vi "SEC code V4.9.vi"() -> ()   [LabVIEW 2022 SP3]
uses:
  SEC code V3.1/Drivers and Aux files/user.lib/atmcd32d.llb/Shutter_type typedef.ctl
  C:/SEC Software V4.91/EcoChemie.Autolab.Sdk.dll
  EcoChemie.Autolab.Sdk.dll
  SEC code V3.1/Drivers and Aux files/State.ctl
  SEC code V3.1/Drivers and Aux files/SECenumctl.ctl
  SEC code V3.1/Drivers and Aux files/user.lib/atmcd32d.llb/TriggerMode_mode typedef.ctl
  SEC code V3.1/Drivers and Aux files/OSSPEC.ctl
  SEC code V3.1/Drivers and Aux files/OSPEC-enum.ctl
  Labview/IVIUM/IVIUM_remdriver.lvlib
panel:
  out "Current PD 2":dbl
  out "POtential PD 2":dbl
  in  "Tab Control 5":enum32{"AUTOLAB", "IVIUM", "iDUS", "Kymera"}(tab)
  out "current":dbl
  out "Error after autolab connection?":errorcluster
  out "Autolab Connected?":bool
  out "Voltage":dbl format="%#_3e"
  out "PotentialOverload":bool
  out "Bandwidth":i32
  out "CurrentRange":i32
  out "Mode":i32
  out "Measured voltage":dbl
  out "CurrentOverload":bool
  out "Cell on?":bool
  out "current":dbl caption="Current (A)" format="%_4g"
  out "cell on":bool
  out "V (during measurment)":dbl
  out "Potentiostat Status":string
  out "T reached?":bool
  out "Shut down sequence run?":bool
  out "Curent Temp":i32
  in  "Tab Control 4":T1(tab)
  in  "Use autolab?":bool=TRUE
  in  "Embedded Exe File":path=path "C:/Program Files/Metrohm Autolab/Autolab SDK 2.1/Hardware Setup Files/Adk.x"
  in  "Hardware Setup File":path=path "C:/ProgramData/Metrohm Autolab/13.0/HardwareSetup.AUT55444.xml"
  in  "Bandwidth 2":i32(ring)=2 items=["UltraHigh_Speed", "High_Speed", "High_Stability"]
  in  "Start potential (V)":dbl=0.2
  in  "Stop potential (V)":dbl=0.7
  in  "Increment (V)":dbl=0.05
  in  "Default Potential (V)":dbl=0.2
  in  "Wait before \nspectrum (s)":dbl=0.1
  in  "Equilibration \ntime (s)":u32=5
  in  "Reverse Scan\ndirection":bool
  in  "(update and read)":bool
  in  "Tab Control 3":T2(tab)=enum."iDUS run"
  in  "Inetegration\n Time (us)":i32=8000
  in  "Continuous \nStrobe Delay (us)":i32
  in  "Number of averages":i32
  in  "Use iDus?":bool
  in  "Return detector \nto room T?":bool
  in  "Init, Cool, read dark,\nOR\nWarm/de-init detector":bool
  in  "Temperature\n(degrees C)":i32=-80
  in  "Number of scans in kinetic cycle":i32=30
  in  "Exposure time (s)":dbl=0.03
  in  "Tab Control 2":T3(tab)
  in  "V 1 time (s)":dbl=10.0
  in  "V off time":dbl=30.0
  in  "Sampling\n delay (s)":dbl
  in  "V 2 time (s)":dbl=20.0
  in  "Run OSPSEC":bool
  in  "Square wave?":bool
  out "OCP I (close to 0)":dbl
  out "OCP":dbl format="%_3f"
  in  "V1 (V)":dbl=0.4
  in  "V2 (V)":dbl=0.8
  in  "Slow sample time (s)":dbl=1500.0
  out "Time during PD":u32
  in  "File Name":string="test-1"
  in  "File Path":path=path "C:/Data"
  in  "Tab Control":T4(tab)
  out "?":T5(graph)
  out "?":cluster{i32[], dbl[]}(graph)
  out "?":T5(graph)
  out "?":T5(graph)
  out "Current during PD":dbl(graph)=1.602783203125e-06
  out "?":cluster{dbl[], dbl[]}(graph)
  out "Potential  During PD":dbl(graph)=-0.0002471923828124972
  out "Setpoint":dbl
  out "?":cluster{i32[], "array":i32[]}(graph)
  out "I_overload":bool
  out "Aninput1_overload":bool
  out "E_overload":bool
  out "cell-off button pressed":bool
  in  "Default\nCurrent range":T6(ring)=enum."100 uA"
  in  "Default Filter":T7(ring)=enum."10 kHz"
  out "Device serial number":string
  in  "Set Stability":T8(ring)=enum."Standard"
  out "Number of Spectrometers":i32
  out "IDus not in read loop? (kinetic)":bool
  out "Get status return code":dbl
  out "xpixels":i32
  out "ypixels":i32
  out "Calculated exposure time":sgl format="%.2f"
  out "Check timings return code":u32
  out "Set temprature\nreturn code":u32
  out "get aquired data return code":u32
  out "Start Aquisition return code":u32
  out "Init. return code":u32
  out "Cooler Off return code":u32
  out "Time before the start of current aquisition (ms)":u32
  out "Time  after the aquisition (before fetch data), (ms)":u32
  in  "Shutter opens on TTL":T9=enum."TTL High"
  in  "Shutter open and close time":i32
  out "Get aqisition ok? (kinetic mode)":bool
  out "Time taken to apply V2":u32
  out "Values to re-intialise to at end\nof the measument":T10
  out "V2 applied?":bool
  out "ContinuousStrobe Out":u32
  out "Wrapper Out":u32
  out "WL Values":dbl[](array[numeric])
  out "Number of time the OCEAN averaging loop has run -1":i32
  out "Adc":refnum<k24>
  out "Sampler 2":refnum<k24>
  out "Dio":refnum<k24>
  out "Dac":refnum<k24>
  out "instrument":refnum<k24>
  out "Ei":refnum<k24>
  out "AutolabConnection":refnum<k24>
  out "EI status supported for":string[](array[string])
  out "TemperatureOverload":bool
  out "ManualCellSwitch":bool
  out "Oscillation":bool
  out "PD ENDED\nEXIT MEASURMENT":bool=TRUE
  out "Current PD":dbl
  out "POtential PD":dbl
  in  "Exit and disconnect":bool
  # "Program control"
  # "Potential decay control"
  # "Spectrometer control"
  # "System status"
  # "SEC control"
  # "Cell on?"
  # "Use the integration time program in the same folder as this program\nto get the optimum value. For kinetic mode the time resolution is limited \nby integration time"
  # "Unless you know what you are doing keep these at 0.03 and 30"
  # "I overload overload"
  # "off button pressed"
  # "Aninput1 overload"
  # "E overload"
  # "OSPEC loop exit"
  # "Checklist for avoiding errors:\n(1) Light on the IVIUM should be blue with red flashes\nIf the system crahes and the light is red then connect and disconnect in IVUM soft/turn stat off/on\n(2) Maya Pro should read in ocean view/or the get intensity program\nIf maya is not reading connect and disconnect USB.\n(3) If errors persist rrepeat steps 1 + 2 then re-compile code by clicking the\nwhite (run) whilst holding down CRTL + (left) SHIFT\n(4) IF USING THE iDus DO NOT EXIT WITHOUT WARMING CAMERA BACK TO ROOM T,YOU \nWILL DAMAGE IT \n(6) if the IVIUM.dll does not load click broken arrows and \"show error\" until you see the call library function (see blue circles). Double click on this and paste the following into the directory (red circle):   \n%windir%\\Labview\\IVIUM\\IVIUM_remdriver.dll"
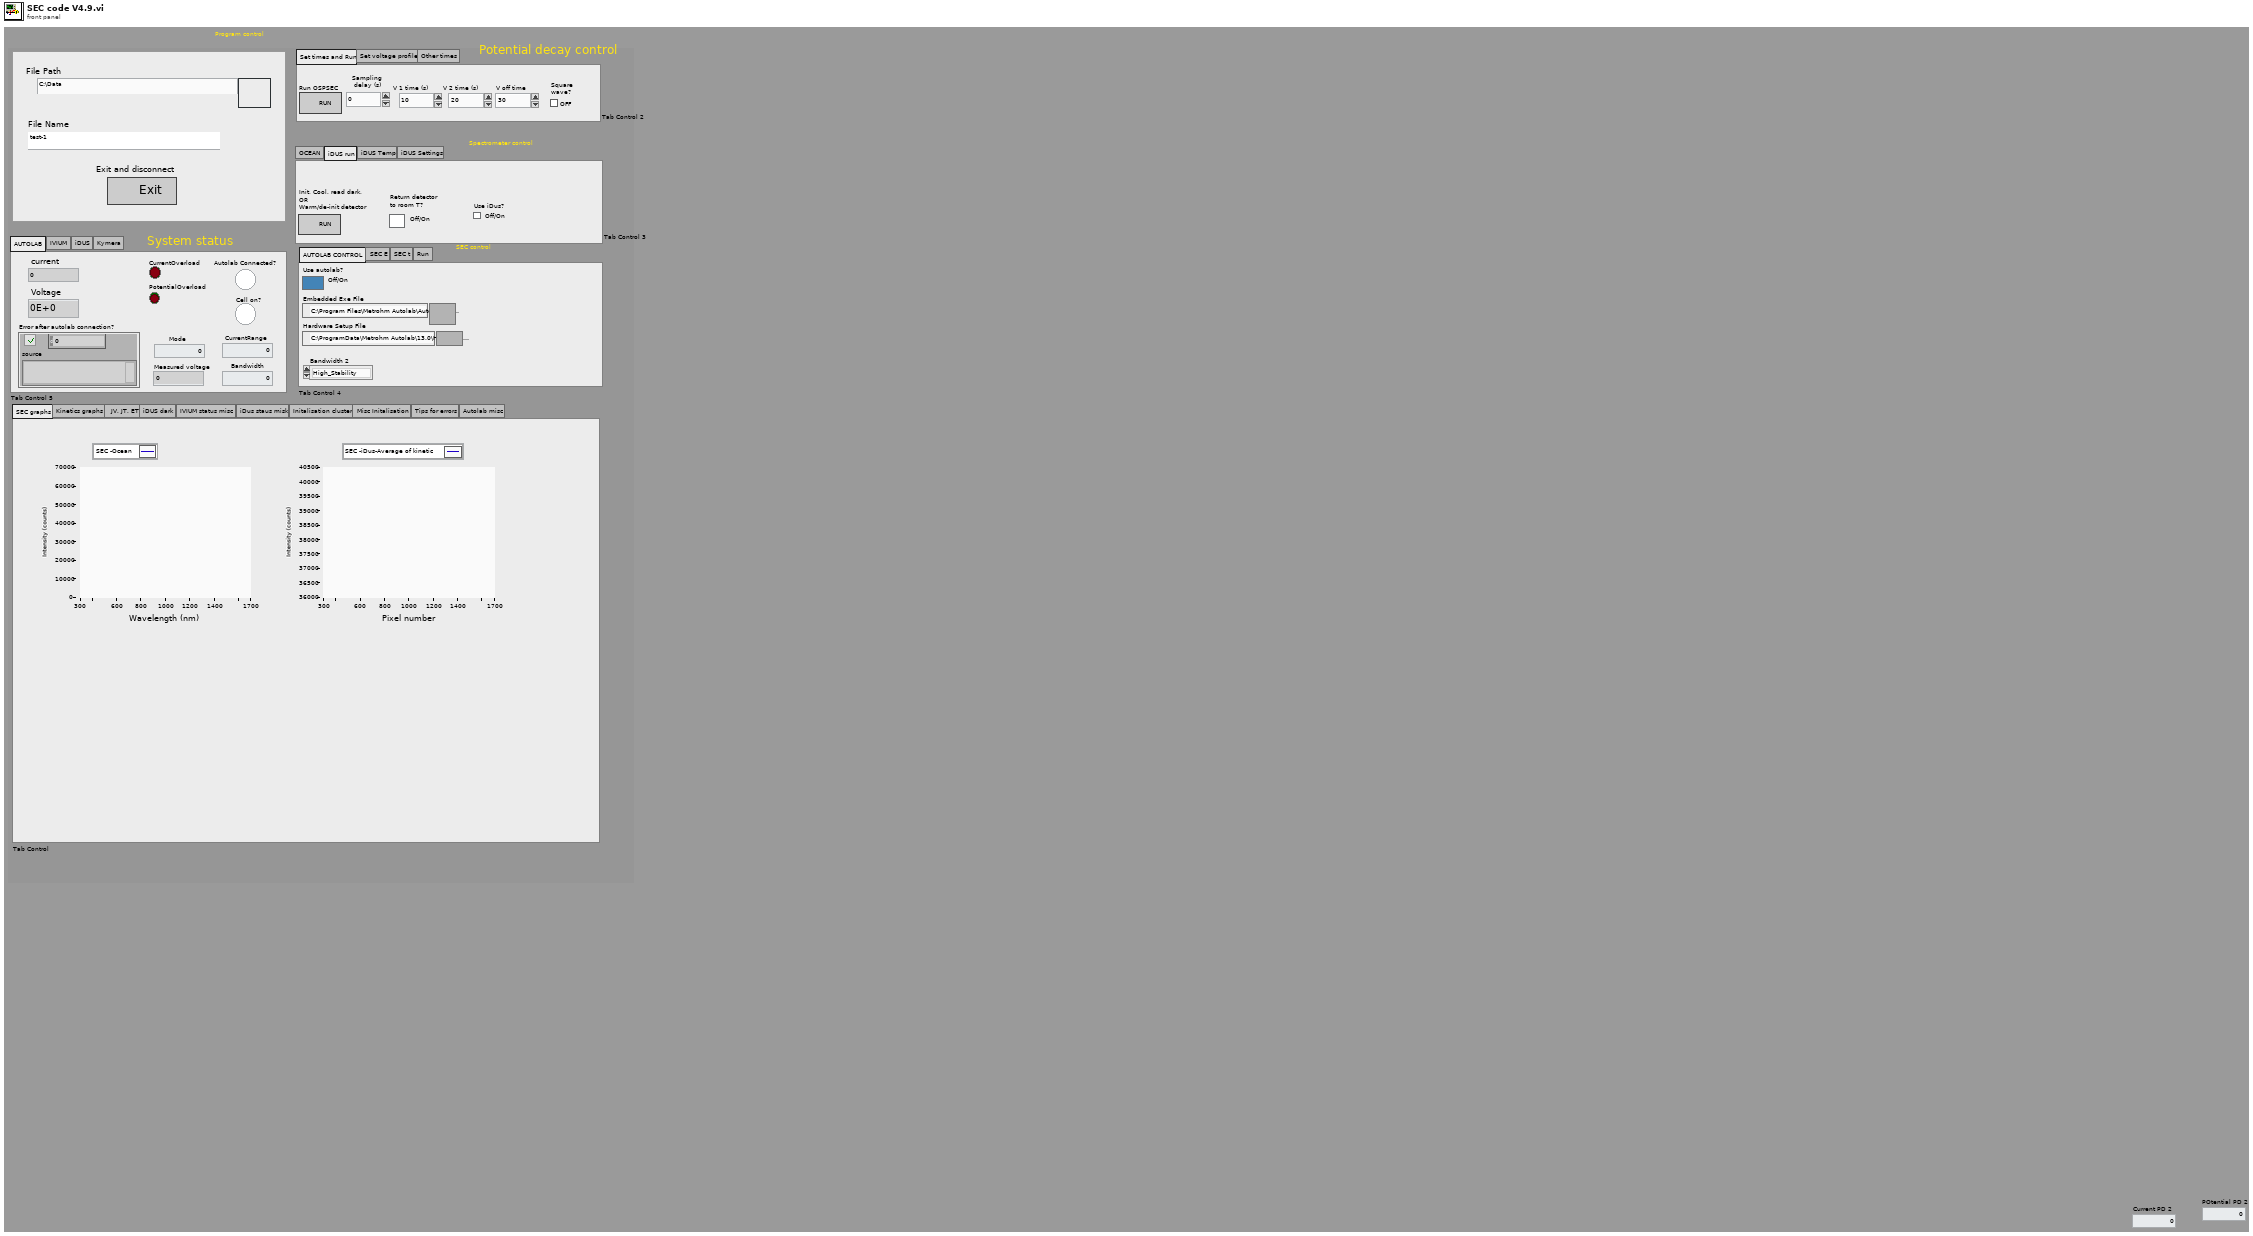
[diagram p1: front panel]
types:
  T1 = enum32{"AUTOLAB CONTROL", "SEC E", "SEC t", "Run"}
  T2 = enum32{"OCEAN", "iDUS run", "iDUS Temp", "iDUS Settings"}
  T3 = enum32{"Set times and Run", "Set voltage profile", "Other times"}
  T4 = enum32{"SEC graphs", "Kinetics graphs", " JV, JT, ET", "iDUS dark", "IVIUM status misc", "iDus staus misk", "Initalisation cluster", "Misc Initalisation ", "Tips for errors", "Autolab misc"}
  T5 = cluster{"WL Values":dbl[], "Spectrum Values":dbl[]}
  T6 = enum16{"10 A", "1 A", "100 mA", "10 mA", "1 mA", "100 uA", "10 uA", "1 uA", "100 nA", "10 nA", "1 nA", "100 pA", "10 pA", "1 pA"}
  T7 = enum16{"1 MHz", "100 kHz", "10 kHz", "1 kHz", "10 Hz"}
  T8 = enum16{"High Speed", "Standard", "High Stability"}
  T9 = typedef "Shutter_type typedef.ctl" = enum16{"TTL Low", "TTL High"}
  T10 = cluster{"Currents":dbl[], "Potentials":dbl[], "Device Status":string, "Device serial no":string, "Current":dbl, "Default \nPotential":dbl, "I overload":bool, "Cell On":bool, "E overload":bool, "Aninput1 overload":bool, "Cell off button pressed":bool, "Start potential":dbl, "Stop potential":dbl, "Increment":dbl, "SEC":dbl[], "Path":path, "File name":string}
  T11 = cluster{"Current array":dbl[], "Potential array":dbl[], "Status":string, "Serial No":string, "Current":dbl, "Default\n potential":dbl, "I overload":bool, "Cell on":bool, "E overload":bool, "Cell of button pressed":bool, "Aninput1 overload":bool, "Stop \npotential":dbl, "Start \npotential":dbl, "Increment":dbl, "Spectrum":dbl[][], "Path":path, "File Name":string, "Sample rate":dbl, "V2 time":dbl, "V off time":dbl, "V 2":dbl, "V 1":dbl, "V1 time":dbl, "Time array":dbl[], "Integration time":i32, "Continous strobe delay":i32, "Time elapsed ":i32, "Start time":i32, "Time for E measurment":i32[], "Time for I measurment ":i32[], "Time for spectrum measurment":i32[], "Return detector to \nroom T":bool, "Number of scans in kinetic cycle":i32, "Exposure time":dbl}
  T12 = typedef "State.ctl" = enum16{"Initialize", "Wait for Event", "Run SEC", "Run OSPEC", "Initialse and cool iDus", "Exit"}
  T13 = typedef "SECenumctl.ctl" = enum16{"Read spectrum from Ocean", "Read spectrum from iDus", "Apply potential", "Wait", "Apply potential Autolab"}
  T14 = typedef "TriggerMode_mode typedef.ctl" = enum16{"Internal", "External", "N/A (2)", "N/A (3)", "N/A (4)", "N/A (5)", "External Start", "External Exposure (Bulb)", "N/A (8)", "External FVB EM", "Software", "N/A (11)", "External Charge Shifting"}
  T15 = typedef "OSSPEC.ctl" = enum16{"Read Potential and spectrum", "Read current and spectrum", "Reinitialise Cell", "Apply V1", "End measurment", "Apply V2"}
  T16 = typedef "OSPEC-enum.ctl" = enum16{"Check exit", "Read", "Wait"}
  T17 = enum16{"off", "EStat4EL", "EStat2EL", "EStatDummy1", "EStatDummy2", "EStatDummy3", "EStatDummy4", "IStat4EL", "IStat2EL", "IStatDummy", "BiStat4EL", "BiStat2EL"}
  T18 = cluster{"Current array":dbl[], "Potential array":dbl[], "Status":string, "Serial No":string, "Current":dbl, "Default\n potential":dbl, "I overload":bool, "Cell on":bool, "E overload":bool, "Cell of button pressed":bool, "Aninput1 overload":bool, "Stop \npotential":dbl, "Start \npotential":dbl, "Increment":dbl, "Spectrum":dbl[][], "Path":path, "File Name":string, "Sample rate":dbl, "V2 time":dbl, "V off time":dbl, "V 2":dbl, "V 1":dbl, "V1 time":dbl, "Time array":dbl[], "Integration time":i32, "Continous strobe delay":i32, "Time elapsed ":i32, "Start time":i32, "Time for E measurment":i32[], "Time for I measurment ":i32[], "Time for spectrum measurment":i32[], "Return detector to \nroom T":bool, "Number of scans in kinetic cycle":i32, "Exposure time":i32}
  T19 = typedef "Error Code Enum typedef.ctl" = enum32{"N/A (0)", "DRV_ERROR_CODES", "DRV_SUCCESS", "DRV_VXDNOTINSTALLED", "DRV_ERROR_SCAN", "DRV_ERROR_CHECK_SUM", "DRV_ERROR_FILELOAD", "DRV_UNKNOWN_FUNC", "DRV_ERROR_VXD_INIT", "DRV_ERROR_ADDRESS", "DRV_ERROR_PAGELOCK", "DRV_ERROR_PAGEUNLOCK", "DRV_ERROR_BOARDTEST", "DRV_ERROR_ACK", "DRV_ERROR_UP_FIFO", "DRV_ERROR_PATTERN", "N/A (16)", "DRV_ACQUISITION_ERRORS", "DRV_ACQ_BUFFER", "DRV_ACQ_DOWNFIFO_FULL", "DRV_PROC_UNKONWN_INSTRUCTION", "DRV_ILLEGAL_OP_CODE", "DRV_KINETIC_TIME_NOT_MET", "DRV_ACCUM_TIME_NOT_MET", "DRV_NO_NEW_DATA", "N/A (25)", "DRV_SPOOLERROR", "N/A (27)", "N/A (28)", "N/A (29)", "N/A (30)", "N/A (31)", "N/A (32)", "DRV_TEMPERATURE_CODES", "DRV_TEMPERATURE_OFF", "DRV_TEMPERATURE_NOT_STABILIZED", "DRV_TEMPERATURE_STABILIZED", "DRV_TEMPERATURE_NOT_REACHED", "DRV_TEMPERATURE_OUT_RANGE", "DRV_TEMPERATURE_NOT_SUPPORTED", "DRV_TEMPERATURE_DRIFT", "N/A (41)", "N/A (42)", "N/A (43)", "N/A (44)", "N/A (45)", "N/A (46)", "N/A (47)", "N/A (48)", "DRV_GENERAL_ERRORS", "DRV_INVALID_AUX", "DRV_COF_NOTLOADED", "DRV_FPGAPROG", "DRV_FLEXERROR", "DRV_GPIBERROR", "N/A (55)", "N/A (56)", "N/A (57)", "N/A (58)", "N/A (59)", "N/A (60)", "N/A (61)", "N/A (62)", "N/A (63)", "DRV_DATATYPE", "DRV_DRIVER_ERRORS", "DRV_P1INVALID", "DRV_P2INVALID", "DRV_P3INVALID", "DRV_P4INVALID", "DRV_INIERROR", "DRV_COFERROR", "DRV_ACQUIRING", "DRV_IDLE", "DRV_TEMPCYCLE", "DRV_NOT_INITIALIZED", "DRV_P5INVALID", "DRV_P6INVALID", "DRV_INVALID_MODE", "DRV_INVALID_FILTER", "DRV_I2CERRORS", "DRV_I2CDEVNOTFOUND", "DRV_I2CTIMEOUT", "DRV_P7INVALID", "N/A (84)", "N/A (85)", "N/A (86)", "N/A (87)", "N/A (88)", "N/A (89)", "DRV_IOCERROR", "DRV_VRMVERSIONERROR"}
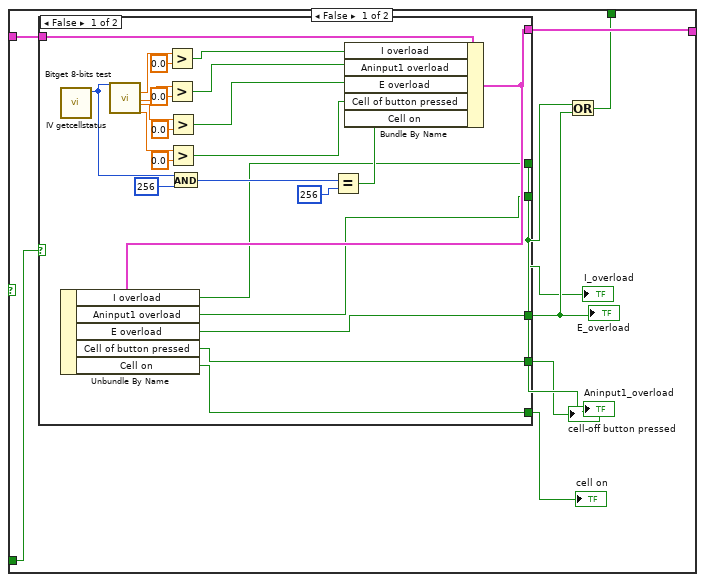
[diagram p2: hidden frame]
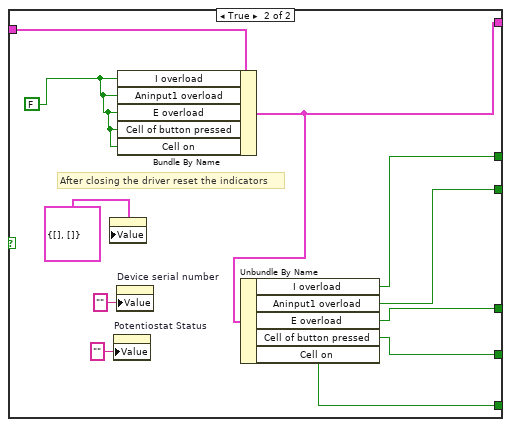
[diagram p3: hidden frame]
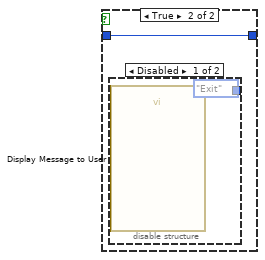
[diagram p4: hidden frame]
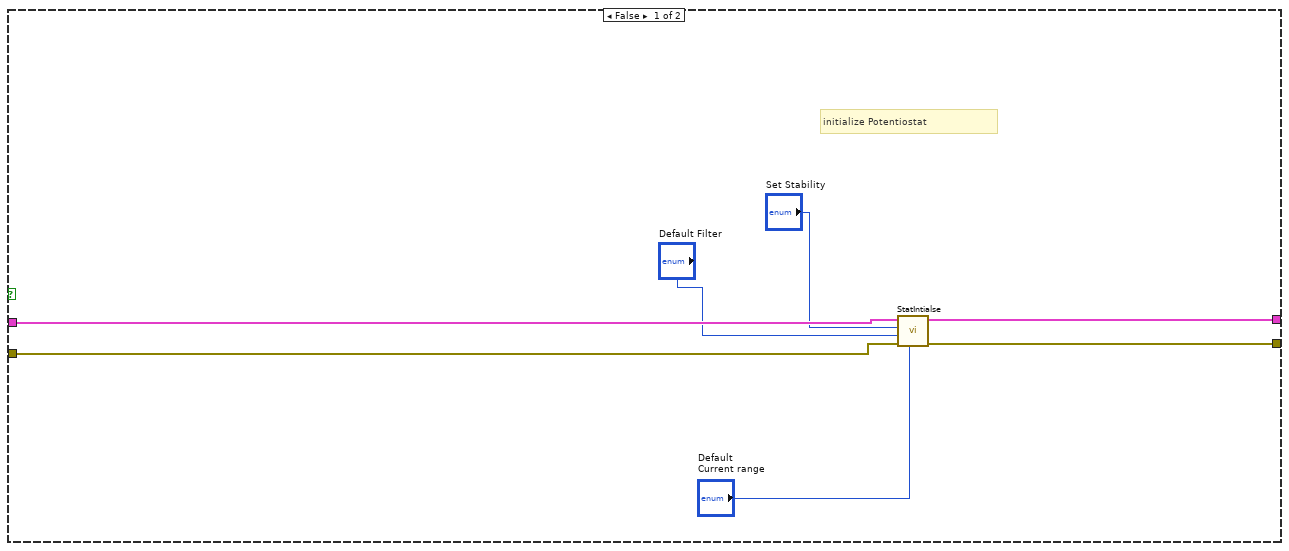
[diagram p7: hidden frame]
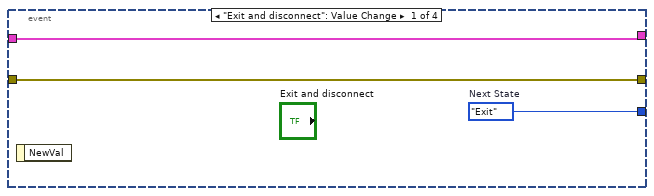
[diagram p9: hidden frame]
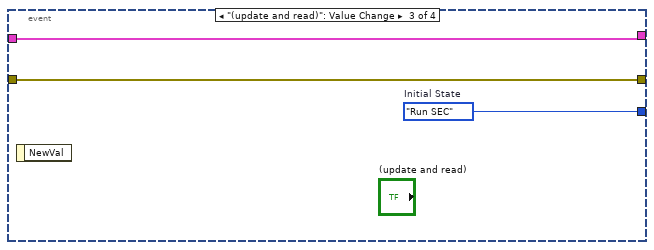
[diagram p10: hidden frame]
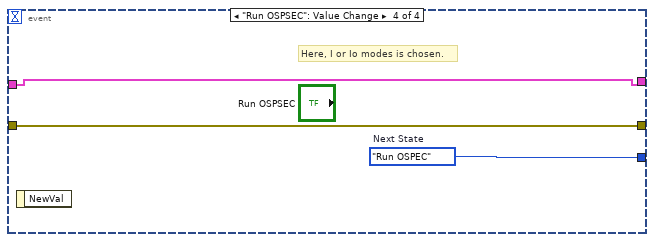
[diagram p11: hidden frame]
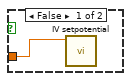
[diagram p13: hidden frame]
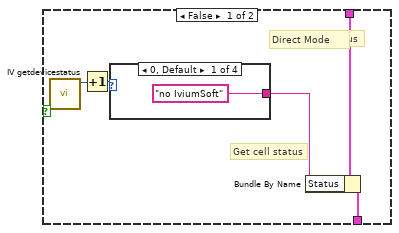
[diagram p14: hidden frame]
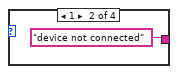
[diagram p15: hidden frame]
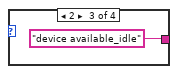
[diagram p16: hidden frame]
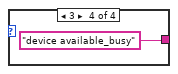
[diagram p17: hidden frame]
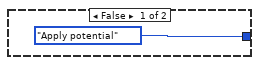
[diagram p18: hidden frame]
diagram:
  w1 = T11 {"Current array"=[], "Potential array"=[], "Status"="", "Serial No"="", "Current"=0.0, "Default\n potential"=0.0, "I overload"=FALSE, "Cell on"=FALSE, "E overload"=FALSE, "Cell of button pressed"=FALSE, "Aninput1 overload"=FALSE, "Stop \npotential"=0.0, "Start \npotential"=0.0, "Increment"=0.0, "Spectrum"=[], "Path"=path "", "File Name"="", "Sample rate"=0.0, "V2 time"=0.0, "V off time"=0.0, "V 2"=0.0, "V 1"=0.0, "V1 time"=0.0, "Time array"=[], "Integration time"=0, "Continous strobe delay"=0, "Time elapsed "=0, "Start time"=0, "Time for E measurment"=[], "Time for I measurment "=[], "Time for spectrum measurment"=[], "Return detector to \nroom T"=FALSE, "Number of scans in kinetic cycle"=0, "Exposure time"=0.0}  # Init cluster
  w3 = State."Initialize"  # Initial State
  n1 = while {
    shift-right: [w21] -> _
    shift-left: w3 -> [w38]
    shift-right: [w24] -> _
    shift-left: w1 -> [w17]
    shift-right: [w25] -> _
    shift-left: errorcluster {"status"=FALSE, "code"=0, "source"=""} ("error constant") -> [w37]
    stop <- w35 stop-if-true
    # "Main VI State Machine"
    n2 = Bundle By Name(cluster=w17, "Sample rate"="Sampling\n delay (s)", "V1 time"="V 1 time (s)", "V2 time"="V 2 time (s)", "V off time"="V off time", "V 2"="V2 (V)", "V 1"="V1 (V)", "Integration time"="Inetegration\n Time (us)", "Continous strobe delay"="Continuous \nStrobe Delay (us)", "Exposure time"="Exposure time (s)", "Number of scans in kinetic cycle"="Number of scans in kinetic cycle") -> (w11:T11)
    n3 = Bundle By Name(cluster=w11, "Default\n potential"="Default Potential (V)", "Start \npotential"="Start potential (V)", "Stop \npotential"="Stop potential (V)", "Increment"="Increment (V)", "Path"="File Path", "File Name"="File Name") -> (w23:T11)
    n4 = case shown="\"Run OSPEC\"" w38 {
      tunnel: [w94 w137 w185 w506 w546 w1742] -> w7
      tunnel: [w93 w134 FALSE ("Stop Loop?") w503 FALSE ("Stop Loop?") _] -> w36
      tunnel: w23 -> [w91 w131 w174 w507 w545 w1740]
      tunnel: [w90 w132 w159 w507 w541 w1740] -> w31
      tunnel: w37 -> [w95 w136 w183 w509 w543 w1739]
      tunnel: [w96 w135 w182 w510 w542 w1739] -> w25
      tunnel: [1 ("devconnect") 1 ("devconnect") 1 ("devconnect") w508 1 ("devconnect") 1 ("devconnect")] -> w22
      frame "Initialize" {
        w93 = FALSE  # Stop Loop?
        w94 = State."Wait for Event"  # Next State
        # "Initialize - Initialize variables needed"
        n5 = case shown="True" "Use autolab?" {
          tunnel: [w104 w109] -> w96
          tunnel: w95 -> [w103 _]
          tunnel: w91 -> [w102 w111]
          tunnel: [w98 w111] -> w90
          frame False {
            # "initialize Potentiostat"
            n6 = call "StatIntialse.vi"("Init cluster 2"=w102, "Set Stability"="Set Stability", "Default\n Filter"="Default Filter", "error in (no error)"=w103, "Default\nCurrent range"="Default\nCurrent range") -> ("Init cluster"=w98:T18, "error out"=w104:errorcluster)  [unwired: 4 in]
          }
          frame True {
            w108 = 2 items=["UltraHigh_Speed", "High_Speed", "High_Stability"] ("Bandwidth")
            w113 = 0 items=["Potentiostatic", "Galvanostatic"] ("Mode")
            w114 = -4 items=["CR07_1A"=0, "CR06_10A"=1, "CR01_100A"=2, "CR00_1000A"=3, "CR05_20A"=20, "CR04_40A"=40, "CR03_50A"=60, "CR02_80A"=80, "CR19_1pA"=-12, "CR18_10pA"=-11, "CR17_100pA"=-10, "CR16_1nA"=-9, "CR15_10nA"=-8, "CR14_100nA"=-7, "CR13_1uA"=-6, "CR12_10uA"=-5, "CR11_100uA"=-4, "CR10_1mA"=-3, "CR09_10mA"=-2, "CR08_100mA"=-1] ("CurrentRange")
            w115 = 1 items=["Off", "On"] ("CellOnOff")
            n7 = call "Connect AutoLab.vi"("Embedded Exe File"="Embedded Exe File", "Hardware Setup File"="Hardware Setup File") -> ("error out"=w120:errorcluster, ".NET Refnum out"=w129:refnum<k24>)  [unwired: 8 in]
            "Error after autolab connection?" <- w120
            n8 = property class="Instrument"(reference=w129, error in=w120) -> (reference out=→"instrument":refnum<k24>, error out=w121:errorcluster, "Adc"=→"Adc":refnum<k24>, "Dac"=→"Dac":refnum<k24>, "Dio"=→"Dio":refnum<k24>, "AutolabConnection"=w117:refnum<k24>, "Ei"=w107:refnum<k24>)
            "AutolabConnection" <- w117
            n9 = property class="AutolabConnection"(reference=w117) -> ("IsConnected"=→"Autolab Connected?":bool)  [unwired: 1 in, 2 out]
            n10 = property class="EI"(reference=w107, error in=w121) -> (reference out=→"Ei":refnum<k24>, error out=w128:errorcluster, "Sampler"=→"Sampler 2":refnum<k24>)
            n11 = Unbundle By Name(w111) -> ("Default\n potential"=w110:dbl)
            n12 = Build Array(w121, w128) -> (w122:errorcluster[])
            n13 = Merge Errors(w122) -> (w112:errorcluster)
            n14 = property class="EI" props=["Bandwidth", "CellOnOff", "CurrentRange", "Mode", "Setpoint", "Current", "Potential", "PotentialApplied", "PotentialOverload", "Sampler", "Setpoint", "PotentialOverload"](reference=w107, error in=w112, "Bandwidth"=w108, "CellOnOff"=w115, "CurrentRange"=w114, "Mode"=w113, "Setpoint"=w110) -> (error out=w109:errorcluster)  [unwired: 8 out]
            n15 = property class="EI"(reference=w107) -> ("Potential"=w106:dbl, "Current"=w105:dbl)  [unwired: 1 in, 2 out]
            n16 = property on="current" class="DigNum (strict)"("Value"=w105) -> ()  [unwired: 2 in, 2 out]
            n17 = property on="Voltage" class="DigNum (strict)"("Value"=w106) -> ()  [unwired: 2 in, 2 out]
          }
        }
        n18 = property on="V2 applied?" class="Bool (strict)"("Value"=FALSE ("V2 applied")) -> ()  [unwired: 2 in, 2 out]
        "Values to re-intialise to at end\nof the measument" <- T10 {"Currents"=[], "Potentials"=[], "Device Status"="", "Device serial no"="", "Current"=0.0, "Default \nPotential"=0.0, "I overload"=FALSE, "Cell On"=FALSE, "E overload"=FALSE, "Aninput1 overload"=FALSE, "Cell off button pressed"=FALSE, "Start potential"=0.0, "Stop potential"=0.0, "Increment"=0.0, "SEC"=[], "Path"=path "", "File name"=""} ("Values to re-intialise to at end\nof the measument")
      }
      frame "Wait for Event" {
        w134 = FALSE  # Stop Loop?
        # "Wait for Event - Use an Event Structure to monitor the user interface for events that run different states of the state machine."
        n19 = event shown="[1] \"Init, Cool, read dark, OR Warm/de-init detector\": Value Change" {
          selector: _ -> [_ _ _ _]
          dyn-events: _ -> [_ _ _ _]
          timeout: _ -> [_ _ _ _]
          tunnel: [w140 State."Initialse and cool iDus" ("Next State") w147 w151] -> w137
          tunnel: w136 -> [w139 w145 w148 w150]
          tunnel: [w139 w145 w148 w150] -> w135
          tunnel: w131 -> [w138 w143 w146 w149]
          tunnel: [w138 w141 w146 w149] -> w132
          event "Exit and disconnect": Value Change {
            w140 = State."Exit"  # Next State
            n20 = event-data() -> ()  [unwired: 1 in, 1 out]
          }
          event "Init, Cool, read dark,\nOR\nWarm/de-init detector": Value Change {
            n21 = event-data() -> ()  [unwired: 1 in, 4 out]
            n22 = Bundle By Name(cluster=w143, "Return detector to \nroom T"="Return detector \nto room T?") -> (w141:T11)
          }
          event "(update and read)": Value Change {
            w147 = State."Run SEC"  # Initial State
            n23 = event-data() -> ()  [unwired: 1 in, 1 out]
          }
          event "Run OSPSEC": Value Change {
            w151 = State."Run OSPEC"  # Next State
            # "Here, I or Io modes is chosen."
            n24 = event-data() -> ()  [unwired: 1 in, 1 out]
          }
        }
      }
      frame "Run SEC" {
        w185 = State."Wait for Event"  # Next State
        n25 = property on="Use autolab?" class="Bool (strict)"() -> ("Value"=w154:bool)  [unwired: 2 in, 2 out]
        n26 = case shown="True" w154 {
          tunnel: w174 -> [w191 w199]
          tunnel: [w190 w199] -> w161
          frame False {
            # "Get cell status"
            # "Get Device Status"
            # "Direct Mode"
            n27 = call "IV getdevicestatus.vi"() -> ("return type"=w193:i32)  [unwired: 10 in, 1 out]
            n28 = Increment(x=w193) -> (x+1=w192:i32)
            n29 = case shown="0, Default" w192 {
              tunnel: ["no IviumSoft" "device not connected" "device available_idle" "device available_busy"] -> w194
              frame 0, Default {
              }
              frame 1 {
              }
              frame 2 {
              }
              frame 3 {
              }
            }
            n30 = Bundle By Name(cluster=w191, "Status"=w194) -> (w190:T11)
          }
          frame True {
          }
        }
        n31 = property on="Use autolab?" class="Bool (strict)"() -> ("Value"=w156:bool)  [unwired: 2 in, 2 out]
        n32 = case shown="True" w156 {
          tunnel: [SECenumctl."Apply potential" SECenumctl."Apply potential Autolab"] -> w181
          frame False {
          }
          frame True {
          }
        }
        n33 = Unbundle By Name(w161) -> ("Increment"=w180:dbl, "Start \npotential"=w184:dbl, "Stop \npotential"=w175:dbl)
        n34 = while {
          shift-right: [w227] -> w158
          shift-left: w161 -> [w228]
          tunnel: w180 -> [w223]
          tunnel: w184 -> [w222]
          shift-right: [w224] -> w182
          shift-left: w183 -> [w225]
          shift-right: [w216] -> _
          shift-left: w181 -> [w220]
          shift-right: [w218] -> w160
          shift-left: dbl[] [0.0] -> [w217]
          shift-right: [w213] -> w164
          shift-left: dbl[] [0.0] -> [w214]
          tunnel: w175 -> [w215]
          shift-right: [w212] -> w173
          shift-left: dbl[][] [] -> [w211]
          tunnel: "Reverse Scan\ndirection" -> [w210]
          tunnel: [w208] -> _
          tunnel: [w208] -> _
          shift-right: [w207] -> _
          shift-left: -3 ("y") -> [w206]
          i -> [w226]
          stop <- w208 stop-if-true
          n35 = case shown="\"Read spectrum from Ocean\"" w220 {
            tunnel: w228 -> [w251 w315 w350 w365 w465]
            tunnel: [w250 w314 w350 w365 w465] -> w227
            tunnel: w226 -> [w264 w324 _ w372 w473]
            tunnel: w225 -> [w261 w306 w346 w374 w474]
            tunnel: [w252 w295 w346 w374 w474] -> w224
            tunnel: w223 -> [w247 w312 _ _ _]
            tunnel: w222 -> [w263 w323 _ _ _]
            tunnel: [w244 w307 w349 w378 w479] -> w221
            tunnel: [w236 w310 w348 w377 w478] -> w219
            tunnel: [w255 w318 w347 w379 w477] -> w218
            tunnel: w217 -> [w256 w319 w347 w379 w477]
            tunnel: [SECenumctl."Wait" SECenumctl."Wait" w351 w360 w461] -> w216
            tunnel: w215 -> [w236 w310 _ _ _]
            tunnel: w214 -> [w254 w317 w342 w380 w475]
            tunnel: [w253 w316 w342 w380 w475] -> w213
            tunnel: [w248 w313 w341 w368 w468] -> w212
            tunnel: w211 -> [w248 w313 w341 w369 w467]
            tunnel: w210 -> [w237 w311 w340 w376 w466]
            tunnel: [w237 w311 w339 w375 w466] -> w209
            tunnel: w206 -> [w235 w305 w337 w362 w462]
            tunnel: [w235 w304 w337 w362 w462] -> w207
            frame "Apply potential", Default {
              # "Here, the while loop iterates three times for every one change of potential. The loop counter is therefore diveded by three, multipled by the increment and then added to the start  potential to give the next potential in the LSV. Potential is applied, then current is read. These go into a build array function . A wait is inclided to alow the sample to equilibriate at the start potential"
              n36 = Divide(x=w264, y=3) -> (x/y=w259:dbl)
              n37 = Multiply(x=w247, y=w259) -> (x*y=w262:dbl)
              n38 = Add(x=w262, y=w263) -> (x+y=w244:dbl)
              "V (during measurment)" <- w244
              n39 = call "IV setpotential.vi"("error in (no error)"=w261, "value"=w244) -> ("error out"=w258:errorcluster)  [unwired: 7 in, 2 out]
              n40 = Equal To 0?(x=w259) -> (x = 0?=w260:bool)
              n41 = case shown="True" w260 {
                tunnel: w258 -> [w274 w276]
                tunnel: [w274 w276] -> w257
                frame False {
                }
                frame True {
                  n42 = Multiply(x=u32 1000, y="Equilibration \ntime (s)") -> (x*y=w275:u32)
                  n43 = Wait (ms)(milliseconds to wait=w275) -> ()  [unwired: 1 out]
                }
              }
              n44 = Equal To 0?(x=w247) -> (x = 0?=w242:bool)
              n45 = Absolute Value(x=w244) -> (abs(x)=w245:dbl)
              n46 = Build Array (concatenate)(w244, w256) -> (w255:dbl[])
              n47 = Greater?(x=w245, y=3.0) -> (0:w243:bool)
              n48 = call "IV getcurrent.vi"("error in (no error)"=w257) -> ("error out"=w240:errorcluster, "value out"=w238:dbl)  [unwired: 8 in, 1 out]
              n49 = Or(x=w242, y=w243) -> (x .or. y?=w241:bool)
              n50 = flat-sequence {
                tunnel: w240 -> [w268]
                tunnel: [w268] -> w239
                tunnel: w238 -> [w267]
                frame #0 {
                  n51 = call "Current ranging routine (SubVI).vi"("Current"=w267) -> ()  [unwired: 11 in]
                  n52 = Wait (ms)(milliseconds to wait=u32 100) -> ()  [unwired: 1 out]
                }
              }
              n53 = case shown="True" w241 {
                frame False {
                }
                frame True {
                  # "abort if E >3 V or\ndelta E =0"
                  n54 = call "IV setcellon.vi"("cellon"=0) -> ("error out"=w272:errorcluster)  [unwired: 8 in, 2 out]
                  n55 = call "IV close.vi"("error in (no error)"=w272) -> ("error out"=w270:errorcluster)  [unwired: 9 in, 1 out]
                  n56 = call "Display Message to User2"("error in (no error)"=w270) -> ("OK"=w273:bool)  [unwired: 9 in, 1 out]
                  n57 = Stop(stop? (T)=w273) -> ()
                }
              }
              n58 = call "IV getcurrent.vi"("error in (no error)"=w239) -> ("error out"=w252:errorcluster, "value out"=w249:dbl)  [unwired: 8 in, 1 out]
              n59 = Bundle By Name(cluster=w251, "Current"=w249) -> (w250:T11)
              n60 = property on="current" class="DigNum (strict)"("Value"=w249) -> ()  [unwired: 2 in, 2 out]
              n61 = Build Array (concatenate)(w249, w254) -> (w253:dbl[])
            }
            frame "Apply potential Autolab" {
              w308 = 1 items=["Off", "On"] ("CellOnOff")
              w303 = 0 items=["Potentiostatic", "Galvanostatic"] ("Mode")
              # "Here, the while loop iterates three times for every one change of potential. The loop counter is therefore diveded by three, multipled by the increment and then added to the start  potential to give the next potential in the LSV. Potential is applied, then current is read. These go into a build array function . A wait is inclided to alow the sample to equilibriate at the start potential"
              n62 = Divide(x=w324, y=3) -> (x/y=w320:dbl)
              n63 = Multiply(x=w312, y=w320) -> (x*y=w322:dbl)
              n64 = Add(x=w322, y=w323) -> (x+y=w307:dbl)
              "Voltage" <- w307
              n65 = property on="Ei" class="Ref (strict)"() -> ("Value"=w282:refnum<k24>)  [unwired: 2 in, 2 out]
              n66 = property class="EI"(reference=w282, error in=w306, "Bandwidth"="Bandwidth 2", "CellOnOff"=w308, "CurrentRange"=w305, "Mode"=w303, "Setpoint"=w307) -> (error out=w287:errorcluster)  [unwired: 1 out]
              n67 = Equal To 0?(x=w320) -> (x = 0?=w321:bool)
              n68 = case shown="True" w321 {
                tunnel: w287 -> [w332 w335]
                tunnel: [w332 w335] -> w299
                frame False {
                }
                frame True {
                  n69 = property on="Equilibration \ntime (s)" class="DigNum (strict)"() -> ("Value"=w333:u32)  [unwired: 2 in, 2 out]
                  n70 = Multiply(x=u32 1000, y=w333) -> (x*y=w334:u32)
                  n71 = Wait (ms)(milliseconds to wait=w334) -> ()  [unwired: 1 out]
                }
              }
              n72 = property on="Sampler 2" class="Ref (strict)"() -> ("Value"=w280:refnum<k24>)  [unwired: 2 in, 2 out]
              n73 = property class="EI"(reference=w282, error in=w287) -> (error out=w286:errorcluster, "EiStatusSupportedFor"=→"EI status supported for":string[])  [unwired: 1 out]
              n74 = invoke class="Sampler" method="Sample"(reference=w280, error in=w287) -> (error out=w285:errorcluster)  [unwired: 1 in, 2 out]
              n75 = Build Array (concatenate)(w307, w319) -> (w318:dbl[])
              n76 = property class="EI"(reference=w282, error in=w299) -> (reference out=w281:refnum<k24>, error out=w298:errorcluster, "Bandwidth"=→"Bandwidth":i32, "CurrentRange"=→"CurrentRange":i32, "Mode"=→"Mode":i32, "Setpoint"=w296:dbl, "Current"=w297:dbl)
              "Measured voltage" <- w296
              n77 = flat-sequence {
                tunnel: w298 -> [w330]
                tunnel: [w330] -> w284
                tunnel: [w329] -> w304
                tunnel: w297 -> [w328]
                tunnel: w296 -> [w327]
                frame #0 {
                  n78 = Wait (ms)(milliseconds to wait=u32 100) -> ()  [unwired: 1 out]
                  n79 = call "Range_selector.vi"("potential"=w327, "current"=w328) -> ("range integer"=w329:i32)  [unwired: 9 in]
                }
              }
              n80 = Merge Errors(w284, w286, w285) -> (w283:errorcluster)
              n81 = call "P_Stat_Status1.vi"("error in (no error)"=w283, ".NET Refnum in"=w281) -> ("error out"=w289:errorcluster, "ManualCellSwitch"=→"ManualCellSwitch":bool, "Oscillation"=→"Oscillation":bool, "TemperatureOverload"=→"TemperatureOverload":bool, "CurrentOverload"=→"CurrentOverload":bool, "Cell"=→"Cell on?":bool)  [unwired: 3 in, 1 out]
              n82 = property class="EI"(reference=w281, error in=w289) -> (error out=w295:errorcluster, "Current"=w279:dbl)  [unwired: 1 out]
              "current" <- w279
              n83 = Bundle By Name(cluster=w315, "Current"=w279) -> (w314:T11)
              n84 = property on="current" class="DigNum (strict)"("Value"=w279) -> ()  [unwired: 2 in, 2 out]
              n85 = Build Array (concatenate)(w279, w317) -> (w316:dbl[])
            }
            frame "Wait" {
              n86 = Multiply(x="Wait before \nspectrum (s)", y=1000.0) -> (x*y=w345:dbl)
              n87 = Wait (ms)(milliseconds to wait=w345) -> ()  [unwired: 1 out]
              n88 = case shown="False" "Use iDus?" {
                tunnel: [SECenumctl."Read spectrum from Ocean" SECenumctl."Read spectrum from iDus"] -> w351
                frame False {
                }
                frame True {
                }
              }
              n89 = case shown="False" w340 {
                selector: w340 -> [w354 w357]
                tunnel: [0.0 1.0] -> w349
                tunnel: [1.0 ("Stop \npotential") 0.0 ("Stop \npotential")] -> w348
                tunnel: [w354 w357] -> w339
                frame False {
                }
                frame True {
                }
              }
            }
            frame "Read spectrum from iDus" {
              n90 = Unbundle By Name(w365) -> ("Exposure time"=w373:dbl, "Number of scans in kinetic cycle"=w366:i32)
              n91 = Equal?(x=w372, y=2) -> (x = y?=w370:bool)
              n92 = Multiply(x=1024, y=w366) -> (x*y=w383:i32)
              n93 = stacked-sequence {
                seq-local: [_ _ _ _ _ _ _ _ _ _ w416 _] -> [_ _ _ _ _ _ _ _ _ _ _ w425]
                tunnel: [_ _ _ _ _ _ _ _ _ _ _ w426] -> w381
                tunnel: w366 -> [_ _ _ _ _ w405 _ _ _ _ _ w424]
                tunnel: w383 -> [_ _ _ _ _ _ _ _ _ _ w417 _]
                tunnel: w373 -> [_ _ _ w401 _ _ _ _ _ _ _ _]
                frame #0 {
                  w398 = u16 3  # AcquisitionMode
                  n94 = call "SetAcquisitionMode.vi"("mode"=w398) -> ()  [unwired: 1 in, 2 out]
                }
                frame #1 {
                  w399 = u16 0  # ReadMode
                  n95 = call "SetReadMode.vi"("mode"=w399) -> ()  [unwired: 1 in, 2 out]
                }
                frame #2 {
                  n96 = call "SetTriggerMode.vi"("mode"=TriggerMode_mode_typedef."Internal") -> ()  [unwired: 1 in, 2 out]
                }
                frame #3 {
                  n97 = call "SetExposureTime.vi"("time"=w401) -> ()  [unwired: 1 in, 2 out]
                }
                frame #4 {
                  n98 = call "GetNumberVSSpeeds.vi"() -> ("number"=w404:i32)  [unwired: 3 in, 2 out]
                  n99 = Subtract(x=w404, y=1) -> (x-y=w402:i32)
                  n100 = call "SetVSSpeed.vi"("index"=w402) -> ()  [unwired: 1 in, 2 out]
                }
                frame #5 {
                  n101 = call "SetNumberKinetics.vi"("number"=w405) -> ()  [unwired: 1 in, 2 out]
                }
                frame #6 {
                  w409 = 0  # Auto Shutter
                  n102 = call "SetShutter.vi"("type"=Shutter_type_typedef."TTL High", "mode"=w409, "closingtime"=0, "openingtime"=0) -> ()  [unwired: 10 in, 2 out]
                }
                frame #7 {
                  n103 = call "GetAcquisitionTimings.vi"() -> ("exposure"=w410:sgl)  [unwired: 11 in, 4 out]
                  n104 = property on="Calculated exposure time" class="DigNum (strict)"("Value"=w410) -> ()  [unwired: 2 in, 2 out]
                }
                frame #8 {
                  n105 = call "StartAcquisition.vi"() -> ("DLL error code"=w411:u32)  [unwired: 2 in, 1 out]
                  n106 = property on="Start Aquisition return code" class="DigNum (strict)"("Value"=w411) -> ()  [unwired: 2 in, 2 out]
                }
                frame #9 {
                  n107 = while {
                    stop <- w414 continue-if-true
                    w415 = u16 72  # DRV ACQUIRING
                    n108 = call "GetStatus.vi"() -> ("DLL error code"=→"Get status return code":u32, "status"=w413:T19)  [unwired: 3 in, 1 out]
                    n109 = Equal?(x=w413, y=w415) -> (x = y?=w414:bool)
                  }
                }
                frame #10 {
                  n110 = flat-sequence {
                    tunnel: [w419] -> w418
                    tunnel: w417 -> [w419]
                    tunnel: [w423] -> w416
                    tunnel: w418 -> [w421]
                    frame #0 {
                    }
                    frame #1 {
                      n111 = call "GetAcquiredData.vi"("size"=w421) -> ("DLL error code"=w420:u32, "array"=w423:i32[])  [unwired: 2 in, 1 out]
                      n112 = Equal?(x=20002 ("DRV_SUCCESS"), y=w420) -> ()  [unwired: 1 out]
                      n113 = property on="get aquired data return code" class="DigNum (strict)"("Value"=w420) -> ()  [unwired: 2 in, 2 out]
                    }
                  }
                }
                frame #11 {
                  n114 = for {
                    N: w424 -> [_]
                    shift-right: [w428] -> w426
                    shift-left: i32[][] [] -> [w430]
                    tunnel: w425 -> [w429]
                    i -> [w433]
                    w431 = 1024 ("x")
                    n115 = Multiply(x=w431, y=w433) -> (x*y=w435:i32)
                    n116 = Equal To 0?(x=w433) -> (x = 0?=w434:bool)
                    n117 = Array Subset(array=w429, index=w435, length=w431) -> (w432:i32[])
                    n118 = case shown="False" w434 {
                      tunnel: w432 -> [w437 w440]
                      tunnel: w430 -> [w438 _]
                      tunnel: [w436 w439] -> w428
                      frame False {
                        n119 = Build Array (concatenate)(w438, w437) -> (w436:i32[][])
                      }
                      frame True {
                        n120 = Build Array(w440) -> (w439:i32[][])
                      }
                    }
                  }
                }
              }
              n121 = property on="Use autolab?" class="Bool (strict)"() -> ("Value"=w361:bool)  [unwired: 2 in, 2 out]
              n122 = case shown="True" w361 {
                tunnel: [SECenumctl."Apply potential" SECenumctl."Apply potential Autolab"] -> w360
                frame False {
                }
                frame True {
                }
              }
              n123 = Unbundle By Name(w365) -> ("Number of scans in kinetic cycle"=w367:i32)
              n124 = flat-sequence {
                tunnel: [w446] -> w363
                tunnel: w381 -> [w444]
                tunnel: w367 -> [w443]
                tunnel: [w441] -> w364
                frame #0 {
                  n125 = for {
                    N: 1023 -> [_]
                    tunnel: w444 -> [w451]
                    tunnel: [w452] -> w446 mode=indexing
                    tunnel: w443 -> [w449]
                    tunnel: [w447] -> w441 mode=indexing
                    i -> [w448]
                    n126 = Index Array(array=w451, index (col)=w448) -> (element=w450:i32[])  [unwired: 1 in]
                    n127 = Add Array Elements(numeric array=w450) -> (sum=w453:i32)
                    n128 = Increment(x=w448) -> (x+1=w447:i32)
                    n129 = Divide(x=w453, y=w449) -> (x/y=w452:dbl)
                  }
                  n130 = Bundle(w441, w446) -> (→"?":cluster{i32[], dbl[]})  [unwired: 1 in]
                }
              }
              n131 = case shown="True" w370 {
                tunnel: w369 -> [w388 _]
                tunnel: w363 -> [w387 w390]
                tunnel: [w386 w391] -> w368
                tunnel: w364 -> [_ w389]
                frame False {
                  n132 = Build Array (concatenate)(w388, w387) -> (w386:dbl[][])
                }
                frame True {
                  n133 = Build Array(w389, w390) -> (w391:dbl[][])
                }
              }
              n134 = case shown="False" w376 {
                selector: w376 -> [w392 w395]
                tunnel: [0.0 1.0] -> w378
                tunnel: [1.0 ("Stop \npotential") 0.0 ("Stop \npotential")] -> w377
                tunnel: [w392 w395] -> w375
                frame False {
                }
                frame True {
                }
              }
            }
            frame "Read spectrum from Ocean" {
              # "Building an matric of WL + intensities of multiple expts"
              n135 = Unbundle By Name(w465) -> ("Integration time"=w464:i32, "Continous strobe delay"=w463:i32)
              n136 = Initialize Array(0.0 ("element"), 2061 ("dimension size")) -> (w454:dbl[])
              n137 = Equal?(x=w473, y=2) -> (x = y?=w471:bool)
              n138 = for {
                N: "Number of averages" -> [_]
                tunnel: [w487] -> w476
                tunnel: [w486] -> w470
                tunnel: w464 -> [w485]
                tunnel: w463 -> [w484]
                shift-right: [w481] -> w459
                shift-left: w454 -> [w482]
                i -> [w480]
                n139 = call "ReadSpectrum(SubVI).vi"("Continuous \nStrobe Delay"=w484, "Enter the \nInetegration Time"=w485) -> ("Spectrum Values"=w483:dbl[], "WL Values"=w486:dbl[], "Number of Spectrometers"=w487:i32)  [unwired: 7 in]
                n140 = Add(x=w483, y=w482) -> (x+y=w481:dbl[])
                "Number of time the OCEAN averaging loop has run -1" <- w480
              }
              "Number of Spectrometers" <- w476
              n141 = Divide(x=w459, y="Number of averages") -> (x/y=w458:dbl[])
              n142 = case shown="False" w471 {
                tunnel: w470 -> [_ w499]
                tunnel: w458 -> [w495 w498]
                tunnel: [w494 w497] -> w468
                tunnel: w467 -> [w496 _]
                frame False {
                  # "Matrix + int on i >3"
                  n143 = Build Array (concatenate)(w496, w495) -> (w494:dbl[][])
                }
                frame True {
                  # "WL + Int on =3"
                  n144 = Build Array(w499, w498) -> (w497:dbl[][])
                }
              }
              n145 = Bundle("WL Values"=w470, w458) -> (→"?":cluster{"WL Values":dbl[], dbl[]})  [unwired: 1 in]
              n146 = property on="Use autolab?" class="Bool (strict)"() -> ("Value"=w460:bool)  [unwired: 2 in, 2 out]
              n147 = case shown="True" w460 {
                tunnel: [SECenumctl."Apply potential" SECenumctl."Apply potential Autolab"] -> w461
                frame False {
                }
                frame True {
                }
              }
              n148 = case shown="False" w466 {
                tunnel: [0.0 1.0] -> w479
                tunnel: [1.0 ("Stop \npotential") 0.0 ("Stop \npotential")] -> w478
                frame False {
                }
                frame True {
                }
              }
            }
          }
          n149 = case shown="False" w209 {
            tunnel: w221 -> [w231 w233]
            tunnel: w219 -> [w230 w232]
            tunnel: [w229 w234] -> w208
            frame False {
              n150 = Greater Or Equal?(x=w231, y=w230) -> (x >= y?=w229:bool)
            }
            frame True {
              n151 = Less Or Equal?(x=w233, y=w232) -> (x <= y?=w234:bool)
            }
          }
        }
        n152 = Unbundle By Name(w158) -> ("Default\n potential"=w179:dbl)
        n153 = property on="Use autolab?" class="Bool (strict)"() -> ("Value"=w153:bool)  [unwired: 2 in, 2 out]
        n154 = Insert Into Array(array=w160, index=0, new element=0.0 ("new element/subarray")) -> (w169:dbl[])
        n155 = Transpose Matrix(1:w173) -> (0:w172:dbl[][])
        n156 = Bundle(w160, w164) -> (→"?":cluster{dbl[], dbl[]})  [unwired: 1 in]
        n157 = Reverse 1D Array(array=w169) -> (reversed array=w168:dbl[])
        n158 = property on="V (during measurment)" class="DigNum (strict)"("Value"=w179) -> ()  [unwired: 2 in, 2 out]
        n159 = case shown="True" w153 {
          tunnel: w179 -> [w187 w189]
          frame False {
            n160 = call "IV setpotential.vi"("value"=w187) -> ()  [unwired: 8 in, 3 out]
          }
          frame True {
            n161 = property on="Ei" class="Ref (strict)"() -> ("Value"=w188:refnum<k24>)  [unwired: 2 in, 2 out]
            n162 = property class="EI"(reference=w188, "Setpoint"=w189) -> ()  [unwired: 1 in, 2 out]
          }
        }
        n163 = Replace Array Subset(array=w172, new element=w168, index (row)=0 ("index")) -> (w157:dbl[][])  [unwired: 1 in]
        n164 = Bundle By Name(cluster=w158, "Spectrum"=w172, "Current array"=w164, "Potential array"=w160) -> (w159:T11)
        n165 = Build Array(w160, w164) -> (w171:dbl[][])
        n166 = disable-structure shown="Enabled" {
          disable-tunnel: w157 -> [w205 _]
          disable-tunnel: w158 -> [w204 _]
          frame Enabled {
            n167 = call "WriteSEC.vi"("Init cluster"=w204, "Array"=w205) -> ()  [unwired: 10 in]
          }
          frame Disabled {
          }
        }
        n168 = Transpose Matrix(1:w171) -> (0:w170:dbl[][])
        n169 = disable-structure shown="Enabled" {
          disable-tunnel: w170 -> [w203 _]
          disable-tunnel: w159 -> [w202 _]
          frame Enabled {
            n170 = call "Write_JV.vi"("Init cluster"=w202, "Array"=w203) -> ()  [unwired: 10 in]
          }
          frame Disabled {
          }
        }
      }
      frame "Exit" {
        w503 = TRUE  # Stop Loop?
        w506 = State."Exit"  # (Value Not Used)
        # "Switch cell on/off"
        # "Diconnect device and close Ivium remdriver"
        # "Disconnect Ivium device (when connected)\nbefore terminating this VI"
        # "Exit - Exit the application."
        n171 = property on="Shut down sequence run?" class="Bool (strict)"("Value"=FALSE ("Shut down sequence run?")) -> ()  [unwired: 2 in, 2 out]
        n172 = property on="PotentialOverload" class="Bool (strict)"("Value"=FALSE ("PotentialOverload")) -> ()  [unwired: 2 in, 2 out]
        n173 = property on="T reached?" class="Bool (strict)"("Value"=FALSE ("T reached?")) -> ()  [unwired: 2 in, 2 out]
        n174 = property on="Use autolab?" class="Bool (strict)"() -> ("Value"=w504:bool)  [unwired: 2 in, 2 out]
        n175 = case shown="True" w504 {
          tunnel: [w518 w536] -> w510
          tunnel: w509 -> [w515 w531]
          tunnel: [w513 0 ("devconnect")] -> w508
          frame False {
            w511 = FALSE ("Shut down sequence run?")
            # "This re-initialises a display for the iDus camera"
            # "On"
            # "Close Ivium Driver"
            n176 = To Long Integer(number=0) -> (32bit integer=w517:i32)
            n177 = call "IV setcellon.vi"("error in (no error)"=w515, "cellon"=w517) -> ("error out"=w514:errorcluster)  [unwired: 7 in, 2 out]
            n178 = call "IV getdevicestatus.vi"("error in (no error)"=w514) -> ("error out"=w519:errorcluster, "return type"=w520:i32)  [unwired: 9 in]
            n179 = Greater Than 0?(x=w520) -> (x > 0?=w512:bool)
            n180 = case shown="False" w512 {
              tunnel: [w523 w525] -> w521
              tunnel: w519 -> [w523 _]
              tunnel: [0 ("devconnect") w524] -> w513
              frame False {
              }
              frame True {
                w524 = 0 ("devconnect")
                n181 = call "IV connect.vi"("devconnect"=w524) -> ("error out"=w525:errorcluster)  [unwired: 8 in, 2 out]
              }
            }
            n182 = property on="Shut down sequence run?" class="Bool (strict)"("Value"=w511) -> ()  [unwired: 2 in, 2 out]
            n183 = property on="Return detector \nto room T?" class="Bool (strict)"("Value"=w511) -> ()  [unwired: 2 in, 2 out]
            n184 = call "IV close.vi"("error in (no error)"=w521) -> ("error out"=w518:errorcluster)  [unwired: 9 in, 1 out]
          }
          frame True {
            w530 = 0 items=["Off", "On"] ("CellOnOff")
            n185 = property on="Ei" class="Ref (strict)"() -> ("Value"=w529:refnum<k24>)  [unwired: 2 in, 2 out]
            n186 = property class="EI"(reference=w529, error in=w531, "CellOnOff"=w530) -> (error out=w528:errorcluster)  [unwired: 1 out]
            n187 = property on="ManualCellSwitch" class="Bool (strict)"("Value"=FALSE ("ManualCellSwitch")) -> ()  [unwired: 2 in, 2 out]
            n188 = property on="Cell on?" class="Bool (strict)"("Value"=FALSE ("Cell")) -> ()  [unwired: 2 in, 2 out]
            n189 = property on="instrument" class="Ref (strict)"(error in=w528) -> (error out=w534:errorcluster, "Value"=w535:refnum<k24>)  [unwired: 1 in, 1 out]
            n190 = property on="Autolab Connected?" class="Bool (strict)"("Value"=FALSE ("IsConnected")) -> ()  [unwired: 2 in, 2 out]
            n191 = invoke class="Instrument" method="Disconnect"(reference=w535, error in=w534) -> (error out=w536:errorcluster)  [unwired: 1 in, 2 out]
          }
        }
        n192 = property on="V2 applied?" class="Bool (strict)"("Value"=FALSE ("V2 applied")) -> ()  [unwired: 2 in, 2 out]
      }
      frame "Run OSPEC" {
        n193 = property on="Use autolab?" class="Bool (strict)"() -> ("Value"=w538:bool)  [unwired: 2 in, 2 out]
        n194 = case shown="True" w538 {
          tunnel: w545 -> [w551 w559]
          tunnel: [w550 w559] -> w544
          frame False {
            # "Get cell status"
            # "Get Device Status"
            # "Direct Mode"
            n195 = call "IV getdevicestatus.vi"() -> ("return type"=w554:i32)  [unwired: 10 in, 1 out]
            n196 = Increment(x=w554) -> (x+1=w553:i32)
            n197 = case shown="0, Default" w553 {
              tunnel: ["no IviumSoft" "device not connected" "device available_idle" "device available_busy"] -> w552
              frame 0, Default {
              }
              frame 1 {
              }
              frame 2 {
              }
              frame 3 {
              }
            }
            n198 = Bundle By Name(cluster=w551, "Status"=w552) -> (w550:T11)
          }
          frame True {
          }
        }
        n199 = while {
          shift-right: [w560] -> w542
          shift-left: w543 -> [w565]
          shift-right: [w561] -> w541
          shift-left: w544 -> [w567]
          shift-right: [w564] -> _
          shift-left: OSSPEC."Apply V1" -> [w566]
          i -> [w563]
          stop <- w562 stop-if-true
          n200 = case shown="\"Read current and spectrum\"" w566 {
            tunnel: w567 -> [w571 w960 w1511 w1535 w1597 w1661]
            tunnel: w565 -> [w570 w974 w1515 w1534 w1607 w1689]
            tunnel: [OSSPEC."End measurment" w990 OSSPEC."Read Potential and spectrum" OSSPEC."Read current and spectrum" OSSPEC."Read current and spectrum" OSSPEC."End measurment"] -> w564
            tunnel: [w576 w973 w1514 w1530 w1598 w1687] -> w560
            tunnel: [w577 w981 w1511 w1531 w1597 w1661] -> w561
            tunnel: w563 -> [_ _ _ _ _ _]
            tunnel: [FALSE FALSE FALSE FALSE FALSE w1688] -> w562
            frame "Read Potential and spectrum", Default {
              n201 = property on="Use autolab?" class="Bool (strict)"() -> ("Value"=w568:bool)  [unwired: 2 in, 2 out]
              n202 = disable-structure shown="Enabled" {
                disable-tunnel: w570 -> [w592 _]
                disable-tunnel: [w591 _] -> w569
                disable-tunnel: w568 -> [w590 _]
                frame Enabled {
                  n203 = case shown="True" w590 {
                    tunnel: w592 -> [w594 w606]
                    tunnel: [w593 w604] -> w591
                    frame False {
                      n204 = flat-sequence {
                        tunnel: w594 -> [w597]
                        tunnel: [w597] -> w595
                        tunnel: [w598] -> w593
                        tunnel: w595 -> [w599]
                        frame #0 {
                          n205 = Wait (ms)(milliseconds to wait=u32 50) -> ()  [unwired: 1 out]
                        }
                        frame #1 {
                          n206 = To Long Integer(number=T17."IStat4EL" ("Configuration")) -> (32bit integer=w601:i32)
                          n207 = call "IV setconnectionmode.vi"("error in (no error)"=w599, "value"=w601) -> ("error out"=w598:errorcluster)  [unwired: 7 in, 2 out]
                        }
                      }
                    }
                    frame True {
                      w602 = 0 items=["Off", "On"] ("CellOnOff")
                      w607 = -6 items=["CR07_1A"=0, "CR06_10A"=1, "CR01_100A"=2, "CR00_1000A"=3, "CR05_20A"=20, "CR04_40A"=40, "CR03_50A"=60, "CR02_80A"=80, "CR19_1pA"=-12, "CR18_10pA"=-11, "CR17_100pA"=-10, "CR16_1nA"=-9, "CR15_10nA"=-8, "CR14_100nA"=-7, "CR13_1uA"=-6, "CR12_10uA"=-5, "CR11_100uA"=-4, "CR10_1mA"=-3, "CR09_10mA"=-2, "CR08_100mA"=-1] ("CurrentRange")
                      w608 = 1 items=["Potentiostatic", "Galvanostatic"] ("Mode")
                      n208 = property on="Ei" class="Ref (strict)"() -> ("Value"=w603:refnum<k24>)  [unwired: 2 in, 2 out]
                      n209 = property class="EI"(reference=w603, error in=w606, "CurrentRange"=w607) -> (error out=w605:errorcluster)  [unwired: 1 out]
                      n210 = property class="EI"(reference=w603, error in=w605, "Mode"=w608, "CellOnOff"=w602) -> (error out=w604:errorcluster)  [unwired: 1 out]
                    }
                  }
                }
                frame Disabled {
                }
              }
              n211 = Unbundle By Name(w571) -> ("Spectrum"=w579:dbl[][])
              n212 = Unbundle By Name(w571) -> ("Time for spectrum measurment"=w578:i32[], "Start time"=w581:i32)
              n213 = Unbundle By Name(w571) -> ("Potential array"=w574:dbl[])
              n214 = property on="Use iDus?" class="Bool (strict)"() -> ("Value"=w572:bool)  [unwired: 2 in, 2 out]
              n215 = Unbundle By Name(w571) -> ("Time for E measurment"=w573:i32[], "Start time"=w580:i32)
              n216 = while {
                shift-right: [w840] -> _
                shift-left: w571 -> [w841]
                shift-right: [w832] -> _
                shift-left: OSPEC-enum."Wait" -> [w842]
                shift-right: [w839] -> w584
                shift-left: w573 -> [w838]
                shift-right: [w833] -> w583
                shift-left: w574 -> [w836]
                shift-right: [w835] -> _
                shift-left: w580 -> [w834]
                shift-right: [w830] -> w576
                shift-left: w569 -> [w831]
                i -> [w837]
                stop <- w827 stop-if-true
                n217 = case shown="\"Read\", Default" w842 {
                  tunnel: w841 -> [w850 w861 w952]
                  tunnel: [w850 w861 w952] -> w840
                  tunnel: [w849 FALSE FALSE] -> w829
                  tunnel: [w854 w865 w950] -> w839
                  tunnel: w838 -> [w854 w866 w950]
                  tunnel: w837 -> [_ w870 _]
                  tunnel: [w852 w869 w947] -> w833
                  tunnel: w836 -> [w852 w868 w947]
                  tunnel: [w845 w862 w949] -> w835
                  tunnel: w834 -> [w845 _ w949]
                  tunnel: [OSPEC-enum."Wait" OSPEC-enum."Check exit" OSPEC-enum."Read"] -> w832
                  tunnel: w831 -> [w851 w858 w946]
                  tunnel: [w851 w857 w946] -> w830
                  frame "Check exit" {
                    n218 = Unbundle By Name(w850) -> ("V off time"=w847:dbl)
                    n219 = Multiply(x=w847, y=1000.0) -> (x*y=w848:dbl)
                    n220 = Greater Or Equal?(x=w845, y=w848) -> (x >= y?=w849:bool)
                  }
                  frame "Read", Default {
                    # "Building a 1d matrix of potentials and times"
                    n221 = property on="Use autolab?" class="Bool (strict)"() -> ("Value"=w855:bool)  [unwired: 2 in, 2 out]
                    n222 = case shown="True" w855 {
                      tunnel: [w873 w876] -> w859
                      tunnel: w858 -> [w872 w874]
                      tunnel: [w871 w875] -> w857
                      frame False {
                        n223 = call "IV getpotential.vi"("error in (no error)"=w872) -> ("error out"=w871:errorcluster, "value out"=w873:dbl)  [unwired: 8 in, 1 out]
                      }
                      frame True {
                        n224 = disable-structure shown="Enabled" {
                          disable-tunnel: [w881 _ w927] -> w876
                          disable-tunnel: [w880 _ w929] -> w875
                          disable-tunnel: w874 -> [w878 _ w937]
                          frame Disabled {
                            n225 = property on="Ei" class="Ref (strict)"() -> ("Value"=w879:refnum<k24>)  [unwired: 2 in, 2 out]
                            n226 = disable-structure shown="Enabled" {
                              disable-tunnel: w879 -> [w889 _]
                              disable-tunnel: w878 -> [w885 w890]
                              disable-tunnel: [w884 w890] -> w877
                              frame Disabled {
                                w886 = -4 items=["CR07_1A"=0, "CR06_10A"=1, "CR01_100A"=2, "CR00_1000A"=3, "CR05_20A"=20, "CR04_40A"=40, "CR03_50A"=60, "CR02_80A"=80, "CR19_1pA"=-12, "CR18_10pA"=-11, "CR17_100pA"=-10, "CR16_1nA"=-9, "CR15_10nA"=-8, "CR14_100nA"=-7, "CR13_1uA"=-6, "CR12_10uA"=-5, "CR11_100uA"=-4, "CR10_1mA"=-3, "CR09_10mA"=-2, "CR08_100mA"=-1] ("CurrentRange")
                                w888 = 1 items=["Potentiostatic", "Galvanostatic"] ("Mode")
                                n227 = property class="EI"(reference=w889, error in=w885, "Mode"=w888, "Setpoint"=0.0, "CurrentRange"=w886) -> (error out=w884:errorcluster)  [unwired: 1 out]
                              }
                              frame Enabled {
                              }
                            }
                            n228 = property class="EI"(reference=w879, error in=w877) -> (error out=w880:errorcluster, "Current"=w882:dbl, "Potential"=w881:dbl)  [unwired: 1 out]
                            n229 = disable-structure shown="Enabled" {
                              disable-tunnel: w882 -> [w883 _]
                              frame Disabled {
                                "OCP I (close to 0)" <- w883
                              }
                              frame Enabled {
                              }
                            }
                          }
                          frame Disabled {
                            n230 = property on="Property Node" class="Ref (strict)"() -> ("Value"=w892:refnum<k24>)  [unwired: 2 in, 2 out]
                            n231 = disable-structure shown="Disabled" {
                              disable-tunnel: _ -> [w918 _]
                              disable-tunnel: [w917 _] -> _
                              disable-tunnel: _ -> [w914 _]
                              disable-tunnel: w892 -> [w913 _]
                              frame Disabled {
                                w911 = 2 items=["UltraHigh_Speed", "High_Speed", "High_Stability"] ("Bandwidth")
                                w916 = 1 items=["Off", "On"] ("CellOnOff")
                                w912 = 0 items=["Potentiostatic", "Galvanostatic"] ("Mode")
                                n232 = property on="Property Node" class="Ring (strict)"() -> ("Value"=w915:i32)  [unwired: 2 in, 2 out]
                                n233 = property class="EI"(reference=w913, error in=w914, "Bandwidth"=w911, "CellOnOff"=w916, "CurrentRange"=w915, "Mode"=w912, "Setpoint"=w918) -> (error out=w917:errorcluster)  [unwired: 1 out]
                                n234 = property on="Property Node" class="Ref (strict)"(error in=w917) -> (error out=w910:errorcluster, "Value"=w907:refnum<k24>)  [unwired: 1 in, 1 out]
                                n235 = property class="EI"(reference=w913, error in=w917) -> (error out=w908:errorcluster, "EiStatusSupportedFor"=w909:string[])  [unwired: 1 out]
                                n236 = invoke class="Sampler" method="Sample"(reference=w907, error in=w910) -> ()  [unwired: 1 in, 3 out]
                                n237 = property on="Property Node" class="Arr (strict)"(error in=w908, "Value"=w909) -> ()  [unwired: 1 in, 2 out]
                              }
                              frame Enabled {
                              }
                            }
                            n238 = property class="EI"(reference=w892) -> (error in=w894:errorcluster, error out=w893:errorcluster, "Setpoint"=w891:dbl)  [unwired: 1 out]
                            n239 = property class="EI" props=["Bandwidth", "CurrentRange", "Mode", "Setpoint", "Current", "Potential"](reference=w892, error in=w893) -> (error out=w895:errorcluster, "Bandwidth"=w906:i32, "CurrentRange"=w905:i32, "Mode"=w904:i32, "Current"=w898:dbl, "Potential"=w897:dbl)  [unwired: 2 out]
                            n240 = property on="Property Node" class="Ring (strict)"("Value"=w906) -> ()  [unwired: 2 in, 2 out]
                            n241 = property on="Property Node" class="Ring (strict)"("Value"=w905) -> ()  [unwired: 2 in, 2 out]
                            n242 = property on="Property Node" class="Ring (strict)"("Value"=w904) -> ()  [unwired: 2 in, 2 out]
                            n243 = flat-sequence {
                              tunnel: [w922] -> w903
                              tunnel: w898 -> [w921]
                              tunnel: w897 -> [w920]
                              tunnel: [w919] -> w896
                              tunnel: w895 -> [w919]
                              frame #0 {
                                n244 = call "Range_selector.vi"("potential"=w920, "current"=w921) -> ("range integer"=w922:i32)  [unwired: 9 in]
                              }
                            }
                            n245 = property class="EI"(reference=w892, error in=w896) -> (error out=w902:errorcluster, "Current"=→"Current PD 2":dbl, "Potential"=→"POtential PD 2":dbl)  [unwired: 1 out]
                            n246 = property class="EI"(reference=w892, error in=w902, "CurrentRange"=w903) -> (error out=w901:errorcluster)  [unwired: 1 out]
                          }
                          frame Enabled {
                            w924 = -9 items=["CR07_1A"=0, "CR06_10A"=1, "CR01_100A"=2, "CR00_1000A"=3, "CR05_20A"=20, "CR04_40A"=40, "CR03_50A"=60, "CR02_80A"=80, "CR19_1pA"=-12, "CR18_10pA"=-11, "CR17_100pA"=-10, "CR16_1nA"=-9, "CR15_10nA"=-8, "CR14_100nA"=-7, "CR13_1uA"=-6, "CR12_10uA"=-5, "CR11_100uA"=-4, "CR10_1mA"=-3, "CR09_10mA"=-2, "CR08_100mA"=-1] ("CurrentRange")
                            w934 = -9 items=["CR07_1A"=0, "CR06_10A"=1, "CR01_100A"=2, "CR00_1000A"=3, "CR05_20A"=20, "CR04_40A"=40, "CR03_50A"=60, "CR02_80A"=80, "CR19_1pA"=-12, "CR18_10pA"=-11, "CR17_100pA"=-10, "CR16_1nA"=-9, "CR15_10nA"=-8, "CR14_100nA"=-7, "CR13_1uA"=-6, "CR12_10uA"=-5, "CR11_100uA"=-4, "CR10_1mA"=-3, "CR09_10mA"=-2, "CR08_100mA"=-1] ("CurrentRange")
                            w938 = 0 items=["Off", "On"] ("CellOnOff")
                            w939 = 2 items=["UltraHigh_Speed", "High_Speed", "High_Stability"] ("Bandwidth")
                            w940 = 1 items=["Potentiostatic", "Galvanostatic"] ("Mode")
                            w944 = 1 items=["Potentiostatic", "Galvanostatic"] ("Mode")
                            w926 = 0 items=["Off", "On"] ("CellOnOff")
                            w945 = 2 items=["UltraHigh_Speed", "High_Speed", "High_Stability"] ("Bandwidth")
                            n247 = property on="Ei" class="Ref (strict)"() -> ("Value"=w936:refnum<k24>)  [unwired: 2 in, 2 out]
                            n248 = property on="Sampler 2" class="Ref (strict)"() -> ("Value"=w935:refnum<k24>)  [unwired: 2 in, 2 out]
                            n249 = call "EI (A).vi"("Sampler"=w935, "Ei"=w936, "CellOnOff"=w926, "Setpoint"=0.0, "Bandwidth"=w945, "CurrentRange"=w934, "Mode"=w944, "error in (no error)"=w937, "Disable Sampler"=FALSE) -> ("Cell"=w933:bool, "PotentialOverload"=w932:bool, "Setpoint"=→"Setpoint":dbl, "error out"=w930:errorcluster)  [unwired: 5 in, 10 out]
                            n250 = property on="PotentialOverload" class="Bool (strict)"("Value"=w932) -> ()  [unwired: 2 in, 2 out]
                            n251 = property on="Cell on?" class="Bool (strict)"("Value"=w933) -> ()  [unwired: 2 in, 2 out]
                            n252 = call "Sampler.vi"("error in (no error)"=w937, "Sampler"=w935) -> ("error out"=w942:errorcluster)  [unwired: 7 in, 2 out]
                            n253 = Merge Errors(w942, w930) -> (w943:errorcluster)
                            n254 = call "EI (A).vi"("Sampler"=w935, "Ei"=w936, "CellOnOff"=w938, "Bandwidth"=w939, "CurrentRange"=w924, "Mode"=w940, "error in (no error)"=w943, "Disable Sampler"=FALSE) -> ("Potential"=w927:dbl, "Current"=w928:dbl, "error out"=w929:errorcluster)  [unwired: 6 in, 11 out]
                            "Potential  During PD" <- w927
                            n255 = property on="current" class="DigNum (strict)"("Value"=w928) -> ()  [unwired: 2 in, 2 out]
                            n256 = property on="Voltage" class="DigNum (strict)"("Value"=w927) -> ()  [unwired: 2 in, 2 out]
                          }
                        }
                      }
                    }
                    "OCP" <- w859
                    n257 = Unbundle By Name(w861) -> ("Start time"=w860:i32)
                    n258 = Tick Count (ms)() -> (millisecond timer value=w856:u32)
                    n259 = Subtract(x=w856, y=w860) -> (x-y=w862:u32)
                    n260 = Equal?(x=1, y=w870) -> ()  [unwired: 1 out]
                    n261 = Build Array (concatenate)(w866, w862) -> (w865:u32[])
                    n262 = Build Array (concatenate)(w868, w859) -> (w869:dbl[])
                  }
                  frame "Wait" {
                    n263 = Unbundle By Name(w952) -> ("Sample rate"=w953:dbl)
                    n264 = Multiply(x=w953, y=1000.0) -> (x*y=w955:dbl)
                    n265 = Wait (ms)(milliseconds to wait=w955) -> ()  [unwired: 1 out]
                  }
                }
                n266 = property on="Use iDus?" class="Bool (strict)"() -> ("Value"=w826:bool)  [unwired: 2 in, 2 out]
                n267 = case shown="False" w826 {
                  tunnel: [TRUE ("Value") w844] -> w828
                  frame False {
                  }
                  frame True {
                    n268 = property on="IDus not in read loop? (kinetic)" class="Bool (strict)"() -> ("Value"=w844:bool)  [unwired: 2 in, 2 out]
                  }
                }
                n269 = And(x=w828, y=w829) -> (x .and. y?=w827:bool)
              }
              n270 = case shown="False" w572 {
                tunnel: [w622 w701] -> w586
                tunnel: [w621 w702] -> w585
                tunnel: w581 -> [w620 w708]
                tunnel: w579 -> [w619 w706]
                tunnel: w578 -> [w618 w704]
                tunnel: [w617 w703] -> w575
                tunnel: w571 -> [w616 w707]
                frame False {
                  n271 = disable-structure shown="Enabled" {
                    disable-tunnel: w616 -> [w634 _]
                    disable-tunnel: [w631 w635] -> w615
                    disable-tunnel: [w630 w637] -> w614
                    disable-tunnel: [w629 w636] -> w613
                    frame Disabled {
                      n272 = Unbundle By Name(w634) -> ("Continous strobe delay"=w632:i32, "Integration time"=w633:i32)
                      n273 = call "OSPEC-Open-Ocean.vi"("Integration Time"=w632, "delay"=w633) -> ("WL Values"=w631:dbl[], "Wrapper Out"=w629:u32, "ContinuousStrobe Out"=w630:u32)  [unwired: 7 in]
                    }
                    frame Enabled {
                      n274 = property on="WL Values" class="Arr (strict)"() -> ("Value"=w635:dbl[])  [unwired: 2 in, 2 out]
                      n275 = property on="ContinuousStrobe Out" class="DigNum (strict)"() -> ("Value"=w637:u32)  [unwired: 2 in, 2 out]
                      n276 = property on="Wrapper Out" class="DigNum (strict)"() -> ("Value"=w636:u32)  [unwired: 2 in, 2 out]
                    }
                  }
                  n277 = while {
                    shift-right: [w652] -> _
                    shift-left: w616 -> [w653]
                    shift-right: [w645] -> _
                    shift-left: OSPEC-enum."Read" -> [w654]
                    shift-right: [w650] -> w621
                    shift-left: w618 -> [w649]
                    shift-right: [w644] -> w617
                    shift-left: w619 -> [w648]
                    shift-right: [w647] -> w622
                    shift-left: w620 -> [w641]
                    tunnel: w613 -> [w643]
                    tunnel: [w642] -> w610
                    tunnel: w615 -> [w640]
                    tunnel: [w639] -> w609
                    tunnel: w614 -> [w638]
                    i -> [w646]
                    stop <- w651 stop-if-true
                    n278 = case shown="\"Wait\"" w654 {
                      tunnel: w653 -> [w664 w676 w695]
                      tunnel: [w664 w676 w695] -> w652
                      tunnel: [w663 FALSE FALSE] -> w651
                      tunnel: [w666 w682 w693] -> w650
                      tunnel: w649 -> [w666 w681 w693]
                      tunnel: w646 -> [_ _ _]
                      tunnel: [w662 w677 w689] -> w644
                      tunnel: w648 -> [w662 w680 w689]
                      tunnel: [w655 w673 w686] -> w647
                      tunnel: w641 -> [w655 _ w686]
                      tunnel: [OSPEC-enum."Wait" OSPEC-enum."Check exit" OSPEC-enum."Read"] -> w645
                      tunnel: w643 -> [w660 w667 w690]
                      tunnel: [w661 w672 w691] -> _
                      tunnel: w640 -> [w661 w672 w691]
                      tunnel: [w660 w667 w690] -> w642
                      tunnel: [w657 w670 w684] -> w639
                      tunnel: w638 -> [w657 w670 w684]
                      frame "Check exit" {
                        n279 = Unbundle By Name(w664) -> ("V off time"=w659:dbl)
                        n280 = Multiply(x=w659, y=1000.0) -> (x*y=w656:dbl)
                        n281 = Greater Or Equal?(x=w655, y=w656) -> (x >= y?=w663:bool)
                      }
                      frame "Read", Default {
                        # "Continue 2d matrix of specta"
                        # "Continue to add times to this"
                        n282 = Tick Count (ms)() -> (millisecond timer value=w674:u32)
                        n283 = call "Wrapper_getSpectrum.vi"("Index"=0, "Wrapper"=w667) -> ("Spectrum Values"=w669:dbl[])  [unwired: 1 out]
                        n284 = Unbundle By Name(w676) -> ("Start time"=w675:i32)
                        n285 = Subtract(x=w674, y=w675) -> (x-y=w673:u32)
                        "Time during PD" <- w673
                        n286 = Bundle("Value"=w672, "Spectrum Values"=w669) -> (→"?":cluster{"Value":dbl[], "Spectrum Values":dbl[]})  [unwired: 1 in]
                        n287 = Build Array (concatenate)(w681, w673) -> (w682:u32[])
                        n288 = Build Array (concatenate)(w680, w669) -> (w677:dbl[][])
                      }
                      frame "Wait" {
                        n289 = Unbundle By Name(w695) -> ("Sample rate"=w696:dbl)
                        n290 = Multiply(x=1000.0, y="Slow sample time (s)") -> (x*y=w685:dbl)
                        n291 = Greater?(x=w686, y=w685) -> (0:w683:bool)
                        n292 = case shown="False" w683 {
                          tunnel: w696 -> [w697 _]
                          frame False {
                            n293 = Multiply(x=w697, y=1000.0) -> (x*y=w699:dbl)
                            n294 = Wait (ms)(milliseconds to wait=w699) -> ()  [unwired: 1 out]
                          }
                          frame True {
                            # "slow down read to measure slow decays\nwithout oversampling"
                            n295 = Wait (ms)(milliseconds to wait=u32 500) -> ()  [unwired: 1 out]
                          }
                        }
                      }
                    }
                  }
                  n296 = flat-sequence {
                    tunnel: [w626] -> w612
                    tunnel: [w625] -> w611
                    tunnel: w609 -> [w625]
                    tunnel: w610 -> [w624]
                    tunnel: w612 -> [w628]
                    tunnel: w611 -> [w627]
                    frame #0 {
                      # "Close spectrometers"
                      n297 = call "Wrapper_closeAllSpectrometers.vi"("Wrapper In"=w624) -> ("Wrapper Out"=w626:u32)
                    }
                    frame #1 {
                      # "Destroy \nwrapper \nand strobe"
                      n298 = call "ContinuousStrobe_Destroy.vi"("ContinuousStrobe"=w627) -> ()
                      n299 = call "Wrapper_Destroy.vi"("Wrapper"=w628) -> ()
                    }
                  }
                }
                frame True {
                  n300 = while {
                    shift-right: [w718] -> w701
                    shift-left: w708 -> [w719]
                    shift-right: [w711] -> _
                    shift-left: OSPEC-enum."Wait" -> [w720]
                    shift-right: [w717] -> w702
                    shift-left: w704 -> [w716]
                    shift-right: [w710] -> w703
                    shift-left: w706 -> [w715]
                    shift-right: [w714] -> _
                    shift-left: w707 -> [w713]
                    i -> [w712]
                    stop <- w709 stop-if-true
                    n301 = case shown="\"Wait\"" w720 {
                      tunnel: w719 -> [w722 _ w823]
                      tunnel: [w722 w731 w823] -> w718
                      tunnel: [w728 FALSE FALSE] -> w709
                      tunnel: [w730 w735 w821] -> w717
                      tunnel: w716 -> [w730 w739 w821]
                      tunnel: w712 -> [_ w742 _]
                      tunnel: w715 -> [w723 w738 w817]
                      tunnel: [w729 w733 w819] -> w714
                      tunnel: w713 -> [w729 w733 w819]
                      tunnel: [OSPEC-enum."Wait" OSPEC-enum."Check exit" OSPEC-enum."Read"] -> w711
                      tunnel: [w723 w736 w817] -> w710
                      frame "Check exit" {
                        n302 = Unbundle By Name(w729) -> ("V off time"=w724:dbl)
                        n303 = Multiply(x=w724, y=1000.0) -> (x*y=w725:dbl)
                        n304 = Greater Or Equal?(x=w722, y=w725) -> (x >= y?=w728:bool)
                      }
                      frame "Read", Default {
                        n305 = Unbundle By Name(w733) -> ("Start time"=w732:i32)
                        n306 = property on="Number of scans in kinetic cycle" class="DigNum (strict)"() -> ("Value"=w734:i32)  [unwired: 2 in, 2 out]
                        n307 = Tick Count (ms)() -> (millisecond timer value=w740:u32)
                        n308 = call "GetDetector.vi"() -> ("xpixels"=w741:i32)  [unwired: 4 in, 3 out]
                        n309 = Subtract(x=w740, y=w732) -> (x-y=w731:u32)
                        n310 = Equal?(x=w742, y=1.0) -> (x = y?=w737:bool)
                        n311 = stacked-sequence {
                          seq-local: [_ _ _ _ _ _ _ _ _ _ w776 _] -> [_ _ _ _ _ _ _ _ _ _ _ w796]
                          seq-local: [_ _ _ _ _ _ _ _ w761 _ _ _] -> [_ _ _ _ _ _ _ _ _ _ _ w794]
                          seq-local: [_ _ _ _ _ _ _ _ _ _ w775 _] -> [_ _ _ _ _ _ _ _ _ _ _ w795]
                          tunnel: [_ _ _ _ _ _ _ _ _ _ _ w789] -> w736
                          tunnel: [_ _ _ _ _ _ _ _ _ _ _ w790] -> w735
                          tunnel: w734 -> [_ _ _ _ _ w754 _ _ _ _ _ w788]
                          tunnel: w731 -> [_ _ _ _ _ _ _ _ _ _ _ w791]
                          tunnel: w731 -> [_ _ _ _ _ _ _ _ _ _ _ _]
                          tunnel: w741 -> [_ w747 _ _ _ _ _ _ _ _ _ _]
                          tunnel: w732 -> [_ _ _ _ _ _ _ _ w760 _ w774 _]
                          tunnel: w739 -> [_ _ _ _ _ _ _ _ _ _ _ w787]
                          tunnel: w738 -> [_ _ _ _ _ _ _ _ _ _ _ w786]
                          tunnel: w737 -> [_ _ _ _ _ _ _ _ _ _ _ w785]
                          frame #0 {
                            w746 = u16 3  # AcquisitionMode
                            n312 = call "SetAcquisitionMode.vi"("mode"=w746) -> ()  [unwired: 1 in, 2 out]
                          }
                          frame #1 {
                            w748 = u16 0  # ReadMode
                            n313 = property on="xpixels" class="DigNum (strict)"("Value"=w747) -> ()  [unwired: 2 in, 2 out]
                            n314 = call "SetReadMode.vi"("mode"=w748) -> ()  [unwired: 1 in, 2 out]
                          }
                          frame #2 {
                            n315 = call "SetTriggerMode.vi"("mode"=TriggerMode_mode_typedef."Internal") -> ()  [unwired: 1 in, 2 out]
                          }
                          frame #3 {
                            n316 = property on="Exposure time (s)" class="DigNum (strict)"() -> ("Value"=w750:dbl)  [unwired: 2 in, 2 out]
                            n317 = call "SetExposureTime.vi"("time"=w750) -> ()  [unwired: 1 in, 2 out]
                          }
                          frame #4 {
                            n318 = call "GetNumberVSSpeeds.vi"() -> ("number"=w753:i32)  [unwired: 3 in, 2 out]
                            n319 = Subtract(x=w753, y=1) -> (x-y=w751:i32)
                            n320 = call "SetVSSpeed.vi"("index"=w751) -> ()  [unwired: 1 in, 2 out]
                          }
                          frame #5 {
                            n321 = call "SetNumberKinetics.vi"("number"=w754) -> ()  [unwired: 1 in, 2 out]
                          }
                          frame #6 {
                            w757 = 0  # Auto Shutter
                            n322 = property on="Shutter open and close time" class="DigNum (strict)"() -> ("Value"=w755:i32)  [unwired: 2 in, 2 out]
                            n323 = property on="Shutter opens on TTL" class="Enum (strict)"() -> ("Value"=w756:T9)  [unwired: 2 in, 2 out]
                            n324 = call "SetShutter.vi"("type"=w756, "mode"=w757, "closingtime"=w755, "openingtime"=w755) -> ()  [unwired: 10 in, 2 out]
                          }
                          frame #7 {
                            # "Meybe delete the exposure time insupt here"
                            n325 = property on="Exposure time (s)" class="DigNum (strict)"() -> ("Value"=w759:dbl)  [unwired: 2 in, 2 out]
                            n326 = call "GetAcquisitionTimings.vi"("exposure input"=w759) -> ("exposure"=w758:sgl)  [unwired: 10 in, 4 out]
                            n327 = property on="Calculated exposure time" class="DigNum (strict)"("Value"=w758) -> ()  [unwired: 2 in, 2 out]
                          }
                          frame #8 {
                            n328 = flat-sequence {
                              tunnel: [w762] -> w761
                              tunnel: w760 -> [w763]
                              frame #0 {
                                n329 = Tick Count (ms)() -> (millisecond timer value=w764:u32)
                                n330 = Subtract(x=w764, y=w763) -> (x-y=w762:u32)
                                n331 = property on="Time before the start of current aquisition (ms)" class="DigNum (strict)"("Value"=w762) -> ()  [unwired: 2 in, 2 out]
                              }
                              frame #1 {
                                n332 = call "StartAcquisition.vi"() -> ("DLL error code"=w765:u32)  [unwired: 2 in, 1 out]
                                n333 = property on="Start Aquisition return code" class="DigNum (strict)"("Value"=w765) -> ()  [unwired: 2 in, 2 out]
                              }
                            }
                          }
                          frame #9 {
                            n334 = while {
                              stop <- w769 continue-if-true
                              w770 = u16 72  # DRV ACQUIRING
                              n335 = call "GetStatus.vi"() -> ("DLL error code"=w767:u32, "status"=w768:T19)  [unwired: 3 in, 1 out]
                              n336 = property on="Get status return code" class="DigNum (strict)"("Value"=w767) -> ()  [unwired: 2 in, 2 out]
                              n337 = Equal?(x=w768, y=w770) -> (x = y?=w769:bool)
                              n338 = property on="IDus not in read loop? (kinetic)" class="Bool (strict)"("Value"=FALSE ("IDus not in read loop? (kinetic)")) -> ()  [unwired: 2 in, 2 out]
                            }
                          }
                          frame #10 {
                            n339 = flat-sequence {
                              tunnel: [w777] -> w775
                              tunnel: w774 -> [w778]
                              tunnel: [w784] -> w776
                              tunnel: w773 -> [w781]
                              frame #0 {
                                n340 = Tick Count (ms)() -> (millisecond timer value=w779:u32)
                                n341 = Subtract(x=w779, y=w778) -> (x-y=w777:u32)
                                n342 = property on="Time  after the aquisition (before fetch data), (ms)" class="DigNum (strict)"("Value"=w777) -> ()  [unwired: 2 in, 2 out]
                              }
                              frame #1 {
                                n343 = call "GetAcquiredData.vi"("size"=w781) -> ("DLL error code"=w782:u32, "array"=w784:i32[])  [unwired: 2 in, 1 out]
                                n344 = Equal?(x=20002 ("DRV_SUCCESS"), y=w782) -> (x = y?=w780:bool)
                                n345 = property on="get aquired data return code" class="DigNum (strict)"("Value"=w782) -> ()  [unwired: 2 in, 2 out]
                                n346 = property on="Get aqisition ok? (kinetic mode)" class="Bool (strict)"("Value"=w780) -> ()  [unwired: 2 in, 2 out]
                              }
                            }
                            n347 = property on="Number of scans in kinetic cycle" class="DigNum (strict)"() -> ("Value"=w771:i32)  [unwired: 2 in, 2 out]
                            n348 = Multiply(x=1024.0, y=w771) -> (x*y=w773:dbl)
                          }
                          frame #11 {
                            n349 = Subtract(x=w795, y=w794) -> (x-y=w793:u32)
                            n350 = Divide(x=w793, y=w788) -> (x/y=w792:dbl)
                            n351 = for {
                              N: w788 -> [_]
                              tunnel: w796 -> [w810]
                              tunnel: w792 -> [w808]
                              tunnel: w791 -> [w806]
                              shift-right: [w804] -> w789
                              shift-left: w786 -> [w803]
                              shift-right: [w800] -> w790
                              shift-left: w787 -> [w801]
                              tunnel: w785 -> [_]
                              i -> [w798]
                              w805 = 1024 ("x")
                              n352 = Multiply(x=w798, y=w808) -> (x*y=w807:dbl)
                              n353 = Multiply(x=w805, y=w798) -> (x*y=w809:i32)
                              n354 = Add(x=w807, y=w806) -> (x+y=w802:dbl)
                              n355 = Array Subset(array=w810, index=w809, length=w805) -> (w797:i32[])
                              n356 = Equal To 0?(x=w798) -> (x = 0?=w799:bool)
                              n357 = case shown="True" w799 {
                                tunnel: w797 -> [_ w812]
                                frame False {
                                }
                                frame True {
                                n358 = for {
                                N: 1023 -> [_]
                                tunnel: [w815] -> w813 mode=indexing
                                i -> [w816]
                                n359 = Increment(x=w816) -> (x+1=w815:i32)
                                }
                                n360 = Bundle(w813, w812) -> (w811:cluster{i32[], i32[]})  [unwired: 1 in]
                                n361 = property class="XYGraph (strict)"("Value"=w811) -> ()  [unwired: 2 in, 2 out]
                                }
                              }
                              n362 = Build Array (concatenate)(w803, w797) -> (w804:dbl[][])
                              n363 = Build Array (concatenate)(w801, w802) -> (w800:dbl[])
                            }
                          }
                        }
                      }
                      frame "Wait" {
                        n364 = Unbundle By Name(w819) -> ("Sample rate"=w818:dbl)
                        n365 = Multiply(x=w818, y=1000.0) -> (x*y=w825:dbl)
                        n366 = Wait (ms)(milliseconds to wait=w825) -> ()  [unwired: 1 out]
                      }
                    }
                    n367 = case shown="True" w709 {
                      selector: w709 -> [_ w721]
                      frame False {
                      }
                      frame True {
                        n368 = property on="IDus not in read loop? (kinetic)" class="Bool (strict)"("Value"=w721) -> ()  [unwired: 2 in, 2 out]
                      }
                    }
                  }
                }
              }
              n369 = Bundle By Name(cluster=w571, "Time for spectrum measurment"=w585, "Time elapsed"=w586, "Spectrum"=w575) -> (w582:T11)
              n370 = Bundle By Name(cluster=w582, "Time for E measurment"=w584, "Potential array"=w583) -> (w577:T11)
            }
            frame "Read current and spectrum" {
              n371 = Unbundle By Name(w960) -> ("Time for spectrum measurment"=w972:i32[], "Start time"=w977:i32)
              n372 = Unbundle By Name(w960) -> ("Current array"=w971:dbl[])
              n373 = Unbundle By Name(w960) -> ("Time for I measurment"=w970:i32[], "Start time"=w976:i32)
              n374 = property on="V2 applied?" class="Bool (strict)"() -> ("Value"=w961:bool)  [unwired: 2 in, 2 out]
              n375 = case shown="False" w961 {
                tunnel: w960 -> [w993 w995]
                tunnel: [w992 w994] -> w959
                frame False {
                  n376 = Unbundle By Name(w993) -> ("V 1"=w992:dbl)
                }
                frame True {
                  n377 = Unbundle By Name(w995) -> ("V 2"=w994:dbl)
                }
              }
              n378 = local read "V (during measurment)"() -> (w978:dbl)
              n379 = Unbundle By Name(w960) -> ("V 1"=w979:dbl, "Spectrum"=w975:dbl[][])
              n380 = property on="Square wave?" class="Bool (strict)"() -> ("Value"=w964:bool)  [unwired: 2 in, 2 out]
              n381 = property on="V2 applied?" class="Bool (strict)"() -> ("Value"=w963:bool)  [unwired: 2 in, 2 out]
              n382 = property on="Use iDus?" class="Bool (strict)"() -> ("Value"=w969:bool)  [unwired: 2 in, 2 out]
              n383 = Equal?(x=w978, y=w979) -> (x = y?=w956:bool)
              n384 = And(x=w964, y=w963) -> (x .and. y?=w958:bool)
              n385 = Not(x=w958) -> (.not. x?=w962:bool)
              n386 = And(x=w956, y=w962) -> (x .and. y?=w957:bool)
              n387 = while {
                shift-right: [w1338] -> _
                shift-left: w960 -> [w1339]
                shift-right: [w1330] -> _
                shift-left: OSPEC-enum."Wait" -> [w1340]
                shift-right: [w1337] -> w982
                shift-left: w970 -> [w1336]
                shift-right: [w1331] -> w968
                shift-left: w971 -> [w1334]
                shift-right: [w1333] -> _
                shift-left: w976 -> [w1332]
                tunnel: w957 -> [w1329]
                shift-right: [w1327] -> w973
                shift-left: w974 -> [w1328]
                tunnel: w959 -> [w1323]
                i -> [w1335]
                stop <- w1324 stop-if-true
                n388 = case shown="\"Read\", Default" w1340 {
                  tunnel: w1339 -> [w1354 w1385 w1495]
                  tunnel: [w1353 w1385 w1495] -> w1338
                  tunnel: [w1351 FALSE FALSE] -> w1325
                  tunnel: [w1356 w1393 w1493] -> w1337
                  tunnel: w1336 -> [w1356 w1394 w1493]
                  tunnel: w1335 -> [_ w1399 _]
                  tunnel: [w1348 w1398 w1491] -> w1331
                  tunnel: w1334 -> [w1348 w1397 w1491]
                  tunnel: [w1346 w1386 w1486] -> w1333
                  tunnel: w1332 -> [w1346 _ w1486]
                  tunnel: [OSPEC-enum."Wait" OSPEC-enum."Check exit" OSPEC-enum."Read"] -> w1330
                  tunnel: w1329 -> [_ w1388 _]
                  tunnel: w1328 -> [w1347 w1380 w1490]
                  tunnel: [w1347 w1383 w1490] -> w1327
                  tunnel: w1323 -> [_ w1379 _]
                  frame "Check exit" {
                    n389 = local read "V (during measurment)"() -> (w1350:dbl)
                    n390 = property on="Square wave?" class="Bool (strict)"() -> ("Value"=w1344:bool)  [unwired: 2 in, 2 out]
                    n391 = property on="V2 applied?" class="Bool (strict)"() -> ("Value"=w1345:bool)  [unwired: 2 in, 2 out]
                    n392 = Unbundle By Name(w1354) -> ("V 1"=w1355:dbl)
                    n393 = Equal?(x=w1355, y=w1350) -> (x = y?=w1352:bool)
                    n394 = And(x=w1344, y=w1345) -> (x .and. y?=w1343:bool)
                    n395 = case shown="True" w1352 {
                      tunnel: w1354 -> [w1362 w1366]
                      tunnel: [w1362 w1366] -> w1353
                      tunnel: [w1361 w1365] -> w1351
                      tunnel: w1346 -> [w1360 w1364]
                      tunnel: w1343 -> [_ w1363]
                      frame False {
                        n396 = Unbundle By Name(w1362) -> ("V2 time"=w1358:dbl)
                        n397 = Multiply(x=1000.0, y=w1358) -> (x*y=w1359:dbl)
                        n398 = Greater Or Equal?(x=w1360, y=w1359) -> (x >= y?=w1361:bool)
                      }
                      frame True {
                        n399 = case shown="True" w1363 {
                          tunnel: w1366 -> [w1369 w1378]
                          tunnel: [w1367 w1377] -> w1365
                          tunnel: w1364 -> [w1368 w1376]
                          frame False {
                            n400 = Unbundle By Name(w1369) -> ("V1 time"=w1372:dbl)
                            n401 = Multiply(x=w1372, y=1000.0) -> (x*y=w1371:dbl)
                            n402 = Greater Or Equal?(x=w1368, y=w1371) -> (x >= y?=w1367:bool)
                          }
                          frame True {
                            n403 = Unbundle By Name(w1378) -> ("V off time"=w1374:dbl)
                            n404 = Multiply(x=w1374, y=1000.0) -> (x*y=w1375:dbl)
                            n405 = Greater Or Equal?(x=w1376, y=w1375) -> (x >= y?=w1377:bool)
                          }
                        }
                      }
                    }
                  }
                  frame "Read", Default {
                    # "Building a 1d matrix of currents"
                    n406 = property on="Use autolab?" class="Bool (strict)"() -> ("Value"=w1381:bool)  [unwired: 2 in, 2 out]
                    n407 = case shown="True" w1381 {
                      tunnel: [w1403 w1411] -> w1392
                      tunnel: [w1402 w1412] -> w1383
                      tunnel: w1380 -> [w1401 w1410]
                      tunnel: w1379 -> [_ w1413]
                      tunnel: w1379 -> [_ w1407]
                      tunnel: w1380 -> [_ w1409]
                      tunnel: w1379 -> [_ w1408]
                      frame False {
                        n408 = flat-sequence {
                          tunnel: w1401 -> [w1405]
                          tunnel: [w1404] -> w1400
                          frame #0 {
                            n409 = call "IV getcurrent.vi"("error in (no error)"=w1405) -> ("error out"=w1404:errorcluster, "value out"=w1406:dbl)  [unwired: 8 in, 1 out]
                            n410 = call "Current ranging routine (SubVI).vi"("Current"=w1406) -> ()  [unwired: 11 in]
                          }
                        }
                        n411 = call "IV getcurrent.vi"("error in (no error)"=w1400) -> ("error out"=w1402:errorcluster, "value out"=w1403:dbl)  [unwired: 8 in, 1 out]
                      }
                      frame True {
                        n412 = disable-structure shown="Enabled" {
                          disable-tunnel: w1413 -> [w1431 _]
                          disable-tunnel: [w1425 w1451] -> w1412
                          disable-tunnel: [w1423 w1450] -> w1411
                          disable-tunnel: w1410 -> [w1418 _]
                          disable-tunnel: w1409 -> [w1417 w1466]
                          disable-tunnel: w1408 -> [w1414 _]
                          disable-tunnel: w1407 -> [_ w1469]
                          frame Disabled {
                            n413 = property on="Ei" class="Ref (strict)"() -> ("Value"=w1415:refnum<k24>)  [unwired: 2 in, 2 out]
                            n414 = disable-structure shown="Disabled" {
                              disable-tunnel: w1431 -> [w1443 _]
                              disable-tunnel: [w1442 _] -> _
                              disable-tunnel: w1418 -> [w1439 _]
                              disable-tunnel: w1415 -> [w1438 _]
                              frame Disabled {
                                w1436 = 2 items=["UltraHigh_Speed", "High_Speed", "High_Stability"] ("Bandwidth")
                                w1441 = 1 items=["Off", "On"] ("CellOnOff")
                                w1437 = 0 items=["Potentiostatic", "Galvanostatic"] ("Mode")
                                n415 = property on="CurrentRange" class="DigNum (strict)"() -> ("Value"=w1440:i32)  [unwired: 2 in, 2 out]
                                n416 = property class="EI"(reference=w1438, error in=w1439, "Bandwidth"=w1436, "CellOnOff"=w1441, "CurrentRange"=w1440, "Mode"=w1437, "Setpoint"=w1443) -> (error out=w1442:errorcluster)  [unwired: 1 out]
                                n417 = property on="Sampler 2" class="Ref (strict)"(error in=w1442) -> (error out=w1435:errorcluster, "Value"=w1432:refnum<k24>)  [unwired: 1 in, 1 out]
                                n418 = property class="EI"(reference=w1438, error in=w1442) -> (error out=w1433:errorcluster, "EiStatusSupportedFor"=w1434:string[])  [unwired: 1 out]
                                n419 = invoke class="Sampler" method="Sample"(reference=w1432, error in=w1435) -> ()  [unwired: 1 in, 3 out]
                                n420 = property on="EI status supported for" class="Arr (strict)"(error in=w1433, "Value"=w1434) -> ()  [unwired: 1 in, 2 out]
                              }
                              frame Enabled {
                              }
                            }
                            n421 = property class="EI"(reference=w1415, error in=w1417, "Setpoint"=w1414) -> (error out=w1416:errorcluster)  [unwired: 1 out]
                            n422 = property class="EI" props=["Bandwidth", "CurrentRange", "Mode", "Setpoint", "Current", "Potential"](reference=w1415, error in=w1416) -> (error out=w1419:errorcluster, "Bandwidth"=w1430:i32, "CurrentRange"=w1429:i32, "Mode"=w1428:i32, "Current"=w1422:dbl, "Potential"=w1421:dbl)  [unwired: 2 out]
                            n423 = property on="Bandwidth" class="DigNum (strict)"("Value"=w1430) -> ()  [unwired: 2 in, 2 out]
                            n424 = property on="CurrentRange" class="DigNum (strict)"("Value"=w1429) -> ()  [unwired: 2 in, 2 out]
                            n425 = property on="Mode" class="DigNum (strict)"("Value"=w1428) -> ()  [unwired: 2 in, 2 out]
                            n426 = flat-sequence {
                              tunnel: [w1447] -> w1427
                              tunnel: w1422 -> [w1446]
                              tunnel: w1421 -> [w1445]
                              tunnel: [w1444] -> w1420
                              tunnel: w1419 -> [w1444]
                              frame #0 {
                                n427 = call "Range_selector.vi"("potential"=w1445, "current"=w1446) -> ("range integer"=w1447:i32)  [unwired: 9 in]
                              }
                            }
                            n428 = property class="EI"(reference=w1415, error in=w1420) -> (error out=w1426:errorcluster, "Current"=w1423:dbl, "Potential"=→"POtential PD":dbl)  [unwired: 1 out]
                            "Current PD" <- w1423
                            n429 = property class="EI"(reference=w1415, error in=w1426, "CurrentRange"=w1427) -> (error out=w1425:errorcluster)  [unwired: 1 out]
                          }
                          frame Enabled {
                            w1453 = 0 items=["Potentiostatic", "Galvanostatic"] ("Mode")
                            w1454 = 1 items=["Off", "On"] ("CellOnOff")
                            w1455 = 1 items=["UltraHigh_Speed", "High_Speed", "High_Stability"] ("Bandwidth")
                            w1459 = 1 items=["Off", "On"] ("CellOnOff")
                            w1460 = 1 items=["UltraHigh_Speed", "High_Speed", "High_Stability"] ("Bandwidth")
                            w1461 = 0 items=["Potentiostatic", "Galvanostatic"] ("Mode")
                            w1470 = 0 items=["Potentiostatic", "Galvanostatic"] ("Mode")
                            w1472 = 1 items=["Off", "On"] ("CellOnOff")
                            w1473 = 1 items=["UltraHigh_Speed", "High_Speed", "High_Stability"] ("Bandwidth")
                            n430 = property on="Sampler 2" class="Ref (strict)"() -> ("Value"=w1457:refnum<k24>)  [unwired: 2 in, 2 out]
                            n431 = property on="CurrentRange" class="DigNum (strict)"() -> ("Value"=w1448:i32)  [unwired: 2 in, 2 out]
                            n432 = property on="Ei" class="Ref (strict)"() -> ("Value"=w1456:refnum<k24>)  [unwired: 2 in, 2 out]
                            n433 = call "EI (A).vi"("Sampler"=w1457, "Ei"=w1456, "CellOnOff"=w1472, "Setpoint"=w1469, "Bandwidth"=w1473, "CurrentRange"=w1448, "Mode"=w1470, "error in (no error)"=w1466, "Disable Sampler"=FALSE) -> ("Cell"=w1467:bool, "Bandwidth"=w1468:i32, "error out"=w1465:errorcluster)  [unwired: 5 in, 11 out]
                            n434 = property on="Bandwidth" class="DigNum (strict)"("Value"=w1468) -> ()  [unwired: 2 in, 2 out]
                            n435 = property on="Cell on?" class="Bool (strict)"("Value"=w1467) -> ()  [unwired: 2 in, 2 out]
                            n436 = call "Sampler.vi"("error in (no error)"=w1466, "Sampler"=w1457) -> ("error out"=w1463:errorcluster)  [unwired: 7 in, 2 out]
                            n437 = Merge Errors(w1463, w1465) -> (w1464:errorcluster)
                            n438 = call "EI (A).vi"("Sampler"=w1457, "Ei"=w1456, "CellOnOff"=w1459, "Bandwidth"=w1460, "Mode"=w1461, "error in (no error)"=w1464, "Disable Sampler"=FALSE) -> ("Potential"=w1458:dbl, "Current"=w1450:dbl, "error out"=w1452:errorcluster)  [unwired: 7 in, 11 out]
                            "Current during PD" <- w1450
                            n439 = property on="Voltage" class="DigNum (strict)"("Value"=w1458) -> ()  [unwired: 2 in, 2 out]
                            n440 = property on="current" class="DigNum (strict)"("Value"=w1450) -> ()  [unwired: 2 in, 2 out]
                            n441 = call "Range_selector.vi"("potential"=w1458, "current"=w1450) -> ("range integer"=w1449:i32)  [unwired: 9 in]
                            n442 = call "EI (A).vi"("Sampler"=w1457, "Ei"=w1456, "CellOnOff"=w1454, "Bandwidth"=w1455, "Mode"=w1453, "error in (no error)"=w1452) -> ("error out"=w1451:errorcluster)  [unwired: 8 in, 13 out]
                            n443 = property on="CurrentRange" class="DigNum (strict)"("Value"=w1449) -> ()  [unwired: 2 in, 2 out]
                          }
                        }
                      }
                    }
                    n444 = Unbundle By Name(w1385) -> ("Start time"=w1384:i32)
                    n445 = Tick Count (ms)() -> (millisecond timer value=w1382:u32)
                    n446 = Subtract(x=w1382, y=w1384) -> (x-y=w1395:u32)
                    n447 = Equal?(x=1, y=w1399) -> (x = y?=w1389:bool)
                    n448 = And(x=w1388, y=w1389) -> (x .and. y?=w1387:bool)
                    n449 = case shown="True" w1387 {
                      tunnel: [w1475 w1479] -> w1393
                      tunnel: w1394 -> [w1476 w1477]
                      tunnel: w1395 -> [w1474 w1478]
                      tunnel: [w1474 w1478] -> w1386
                      frame False {
                        n450 = Build Array (concatenate)(w1476, w1474) -> (w1475:u32[])
                      }
                      frame True {
                        n451 = Build Array (concatenate)(w1477, w1478) -> (w1479:u32[])
                      }
                    }
                    n452 = case shown="False" w1387 {
                      tunnel: [w1481 w1483] -> w1398
                      tunnel: w1397 -> [w1482 _]
                      tunnel: w1392 -> [w1480 w1484]
                      frame False {
                        # "Intensity thereafter"
                        n453 = Build Array (concatenate)(w1482, w1480) -> (w1481:dbl[])
                      }
                      frame True {
                        n454 = Build Array(w1484) -> (w1483:dbl[])
                      }
                    }
                  }
                  frame "Wait" {
                    w1488 = 1000.0 ("y")
                    n455 = Unbundle By Name(w1495) -> ("Sample rate"=w1496:dbl)
                    n456 = property on="Slow sample time (s)" class="DigNum (strict)"() -> ("Value"=w1489:dbl)  [unwired: 2 in, 2 out]
                    n457 = Multiply(x=w1488, y=w1489) -> (x*y=w1487:dbl)
                    n458 = Greater?(x=w1486, y=w1487) -> (0:w1485:bool)
                    n459 = case shown="False" w1485 {
                      tunnel: w1488 -> [_ w1498]
                      tunnel: w1496 -> [_ w1497]
                      frame False {
                      }
                      frame True {
                        n460 = Multiply(x=w1497, y=w1498) -> (x*y=w1499:dbl)
                        n461 = Wait (ms)(milliseconds to wait=w1499) -> ()  [unwired: 1 out]
                      }
                    }
                  }
                }
                n462 = property on="Use iDus?" class="Bool (strict)"() -> ("Value"=w1322:bool)  [unwired: 2 in, 2 out]
                n463 = case shown="False" w1322 {
                  tunnel: [TRUE ("Value") w1342] -> w1326
                  frame False {
                  }
                  frame True {
                    n464 = property on="IDus not in read loop? (kinetic)" class="Bool (strict)"() -> ("Value"=w1342:bool)  [unwired: 2 in, 2 out]
                  }
                }
                n465 = And(x=w1326, y=w1325) -> (x .and. y?=w1324:bool)
              }
              n466 = case shown="False" w969 {
                tunnel: [w1017 w1144] -> w985
                tunnel: [w1016 w1146] -> w984
                tunnel: [w1011 w1143] -> w983
                tunnel: w977 -> [w1015 w1145]
                tunnel: w957 -> [w1014 w1149]
                tunnel: w975 -> [w1013 w1150]
                tunnel: w972 -> [w1012 w1148]
                tunnel: w960 -> [w1005 w1147]
                tunnel: w956 -> [w1000 w1142]
                tunnel: w958 -> [_ w1141]
                tunnel: w958 -> [w1002 _]
                tunnel: w956 -> [w999 _]
                tunnel: w956 -> [w996 _]
                frame False {
                  n467 = case shown="True" w1000 {
                    tunnel: w1002 -> [_ w1023]
                    tunnel: w1000 -> [_ w1022]
                    tunnel: [FALSE w1020] -> w1001
                    frame False {
                    }
                    frame True {
                      n468 = And(x=w1022, y=w1023) -> (x .and. y?=w1021:bool)
                      n469 = Not(x=w1021) -> (.not. x?=w1020:bool)
                    }
                  }
                  n470 = case shown="False" w1001 {
                    tunnel: w1005 -> [_ w1043]
                    tunnel: [w1035 w1038] -> w1010
                    tunnel: [w1036 w1039] -> w1008
                    tunnel: [w1037 w1040] -> w1006
                    frame False {
                      n471 = property on="Wrapper Out" class="DigNum (strict)"() -> ("Value"=w1037:u32)  [unwired: 2 in, 2 out]
                      n472 = property on="ContinuousStrobe Out" class="DigNum (strict)"() -> ("Value"=w1036:u32)  [unwired: 2 in, 2 out]
                      n473 = property on="WL Values" class="Arr (strict)"() -> ("Value"=w1035:dbl[])  [unwired: 2 in, 2 out]
                    }
                    frame True {
                      n474 = Unbundle By Name(w1043) -> ("Continous strobe delay"=w1041:i32, "Integration time"=w1042:i32)
                      n475 = call "OSPEC-Open-Ocean.vi"("Integration Time"=w1042, "delay"=w1041) -> ("WL Values"=w1038:dbl[], "Wrapper Out"=w1040:u32, "ContinuousStrobe Out"=w1039:u32)  [unwired: 7 in]
                      "ContinuousStrobe Out" <- w1039
                      "Wrapper Out" <- w1040
                      "WL Values" <- w1038
                    }
                  }
                  n476 = while {
                    shift-right: [w1060] -> _
                    shift-left: w1005 -> [w1061]
                    shift-right: [w1052] -> _
                    shift-left: OSPEC-enum."Wait" -> [w1062]
                    shift-right: [w1058] -> w1011
                    shift-left: w1012 -> [w1057]
                    shift-right: [w1050] -> w1016
                    shift-left: w1013 -> [w1056]
                    shift-right: [w1055] -> w1017
                    shift-left: w1015 -> [w1054]
                    tunnel: w1014 -> [w1051]
                    tunnel: w1010 -> [w1049]
                    tunnel: [w1048] -> w1009
                    tunnel: w1006 -> [w1045]
                    tunnel: w1008 -> [w1046]
                    tunnel: [w1047] -> w1007
                    tunnel: w996 -> [w1044]
                    i -> [w1053]
                    stop <- w1059 stop-if-true
                    n477 = case shown="\"Read\", Default" w1062 {
                      tunnel: w1061 -> [w1072 w1098 w1136]
                      tunnel: [w1071 w1098 w1136] -> w1060
                      tunnel: [w1069 FALSE FALSE] -> w1059
                      tunnel: [w1073 w1112 w1134] -> w1058
                      tunnel: w1057 -> [w1073 w1111 w1134]
                      tunnel: w1053 -> [_ w1106 _]
                      tunnel: [w1066 w1100 w1132] -> w1050
                      tunnel: w1056 -> [w1066 w1110 w1132]
                      tunnel: [w1070 w1101 w1129] -> w1055
                      tunnel: w1054 -> [w1070 _ w1129]
                      tunnel: [OSPEC-enum."Wait" OSPEC-enum."Check exit" OSPEC-enum."Read"] -> w1052
                      tunnel: w1051 -> [w1067 w1105 _]
                      tunnel: w1049 -> [_ w1091 _]
                      tunnel: [w1065 w1095 w1131] -> w1048
                      tunnel: w1046 -> [w1065 w1095 w1131]
                      tunnel: w1045 -> [w1064 w1094 w1130]
                      tunnel: [w1064 w1094 w1130] -> w1047
                      tunnel: w1044 -> [w1063 _ _]
                      frame "Check exit" {
                        n478 = case shown="False" w1067 {
                          tunnel: w1072 -> [w1080 w1090]
                          tunnel: [w1080 w1090] -> w1071
                          tunnel: w1070 -> [w1078 w1088]
                          tunnel: [w1079 w1089] -> w1069
                          tunnel: w1063 -> [w1074 _]
                          frame False {
                            n479 = case shown="False" w1074 {
                              tunnel: w1080 -> [w1082 w1084]
                              tunnel: [w1081 w1083] -> w1077
                              frame False {
                                n480 = Unbundle By Name(w1082) -> ("V2 time"=w1081:dbl)
                              }
                              frame True {
                                n481 = Unbundle By Name(w1084) -> ("V off time"=w1083:dbl)
                              }
                            }
                            n482 = Multiply(x=w1077, y=1000.0) -> (x*y=w1075:dbl)
                            n483 = Greater Or Equal?(x=w1078, y=w1075) -> (x >= y?=w1079:bool)
                          }
                          frame True {
                            n484 = Unbundle By Name(w1090) -> ("V1 time"=w1087:dbl)
                            n485 = Multiply(x=w1087, y=1000.0) -> (x*y=w1085:dbl)
                            n486 = Greater Or Equal?(x=w1088, y=w1085) -> (x >= y?=w1089:bool)
                          }
                        }
                      }
                      frame "Read", Default {
                        # "Check here to see if DIM t + 1 and DIM WL match"
                        n487 = Tick Count (ms)() -> (millisecond timer value=w1096:u32)
                        n488 = call "Wrapper_getSpectrum.vi"("Index"=0, "Wrapper"=w1094) -> ("Spectrum Values"=w1092:dbl[])  [unwired: 1 out]
                        n489 = Unbundle By Name(w1098) -> ("Start time"=w1097:i32)
                        n490 = Subtract(x=w1096, y=w1097) -> (x-y=w1102:u32)
                        n491 = Bundle("WL Values"=w1091, "Spectrum Values"=w1092) -> (→"?":T5)  [unwired: 1 in]
                        n492 = Equal?(x=w1106, y=1.0) -> (x = y?=w1104:bool)
                        n493 = And(x=w1105, y=w1104) -> (x .and. y?=w1103:bool)
                        n494 = case shown="False" w1103 {
                          tunnel: [w1115 w1116] -> w1100
                          tunnel: w1110 -> [w1114 _]
                          tunnel: w1092 -> [w1113 w1118]
                          tunnel: w1091 -> [_ w1117]
                          frame False {
                            # "Intensity thereafter"
                            n495 = Build Array (concatenate)(w1114, w1113) -> (w1115:dbl[][])
                          }
                          frame True {
                            n496 = Build Array(w1117, w1118) -> (w1116:dbl[][])
                          }
                        }
                        n497 = case shown="False" w1103 {
                          tunnel: [w1121 w1124] -> w1112
                          tunnel: w1111 -> [w1120 w1123]
                          tunnel: w1102 -> [w1119 w1122]
                          tunnel: [w1119 w1122] -> w1101
                          frame False {
                            n498 = Build Array (concatenate)(w1120, w1119) -> (w1121:u32[])
                          }
                          frame True {
                            n499 = Build Array (concatenate)(w1123, w1122) -> (w1124:u32[])
                          }
                        }
                      }
                      frame "Wait" {
                        n500 = Unbundle By Name(w1136) -> ("Sample rate"=w1137:dbl)
                        n501 = property on="Slow sample time (s)" class="DigNum (strict)"() -> ("Value"=w1126:dbl)  [unwired: 2 in, 2 out]
                        n502 = Multiply(x=w1126, y=1000.0) -> (x*y=w1125:dbl)
                        n503 = Greater?(x=w1129, y=w1125) -> (0:w1128:bool)
                        n504 = case shown="False" w1128 {
                          tunnel: w1137 -> [_ w1138]
                          frame False {
                          }
                          frame True {
                            n505 = Multiply(x=w1138, y=1000.0) -> (x*y=w1140:dbl)
                            n506 = Wait (ms)(milliseconds to wait=w1140) -> ()  [unwired: 1 out]
                          }
                        }
                      }
                    }
                  }
                  n507 = property on="V2 applied?" class="Bool (strict)"() -> ("Value"=w1003:bool)  [unwired: 2 in, 2 out]
                  n508 = property on="Square wave?" class="Bool (strict)"() -> ("Value"=w1004:bool)  [unwired: 2 in, 2 out]
                  n509 = And(x=w1004, y=w1003) -> (x .and. y?=w998:bool)
                  n510 = And(x=w998, y=w999) -> (x .and. y?=w997:bool)
                  n511 = case shown="True" w997 {
                    tunnel: w1009 -> [w1024 w1026]
                    tunnel: w1007 -> [w1025 w1027]
                    frame False {
                      n512 = property on="Wrapper Out" class="DigNum (strict)"("Value"=w1025) -> ()  [unwired: 2 in, 2 out]
                      n513 = property on="ContinuousStrobe Out" class="DigNum (strict)"("Value"=w1024) -> ()  [unwired: 2 in, 2 out]
                    }
                    frame True {
                      n514 = flat-sequence {
                        tunnel: [w1032] -> w1029
                        tunnel: [w1031] -> w1028
                        tunnel: w1026 -> [w1031]
                        tunnel: w1027 -> [w1030]
                        tunnel: w1029 -> [w1034]
                        tunnel: w1028 -> [w1033]
                        frame #0 {
                          # "Close spectrometers"
                          n515 = call "Wrapper_closeAllSpectrometers.vi"("Wrapper In"=w1030) -> ("Wrapper Out"=w1032:u32)
                        }
                        frame #1 {
                          # "Destroy \nwrapper \nand strobe"
                          n516 = call "ContinuousStrobe_Destroy.vi"("ContinuousStrobe"=w1033) -> ()
                          n517 = call "Wrapper_Destroy.vi"("Wrapper"=w1034) -> ()
                        }
                      }
                    }
                  }
                }
                frame True {
                  n518 = while {
                    shift-right: [w1164] -> w1144
                    shift-left: w1145 -> [w1165]
                    shift-right: [w1157] -> _
                    shift-left: OSPEC-enum."Wait" -> [w1166]
                    shift-right: [w1163] -> w1143
                    shift-left: w1148 -> [w1162]
                    shift-right: [w1155] -> w1146
                    shift-left: w1150 -> [w1161]
                    shift-right: [w1160] -> _
                    shift-left: w1147 -> [w1159]
                    tunnel: w1149 -> [w1156]
                    tunnel: w1142 -> [w1153]
                    tunnel: w1141 -> [w1152]
                    i -> [w1158]
                    stop <- w1154 stop-if-true
                    n519 = case shown="\"Read\", Default" w1166 {
                      tunnel: w1165 -> [w1175 _ w1309]
                      tunnel: [w1174 w1202 w1309] -> w1164
                      tunnel: [w1172 FALSE FALSE] -> w1154
                      tunnel: [w1176 w1203 w1317] -> w1163
                      tunnel: w1162 -> [w1176 w1208 w1317]
                      tunnel: w1158 -> [_ w1212 _]
                      tunnel: w1161 -> [w1170 w1206 w1313]
                      tunnel: [w1173 w1201 w1315] -> w1160
                      tunnel: w1159 -> [w1173 w1201 w1315]
                      tunnel: [OSPEC-enum."Wait" OSPEC-enum."Check exit" OSPEC-enum."Read"] -> w1157
                      tunnel: w1156 -> [_ w1207 _]
                      tunnel: [w1170 w1204 w1313] -> w1155
                      tunnel: w1153 -> [w1169 _ _]
                      tunnel: w1152 -> [w1168 _ _]
                      frame "Check exit" {
                        n520 = case shown="True" w1169 {
                          tunnel: w1175 -> [w1178 w1187]
                          tunnel: [w1178 w1186] -> w1174
                          tunnel: w1173 -> [w1177 w1185]
                          tunnel: [w1179 w1184] -> w1172
                          tunnel: w1168 -> [_ w1183]
                          frame False {
                            n521 = Unbundle By Name(w1177) -> ("V2 time"=w1180:dbl)
                            n522 = Multiply(x=w1180, y=1000.0) -> (x*y=w1181:dbl)
                            n523 = Greater Or Equal?(x=w1178, y=w1181) -> (x >= y?=w1179:bool)
                          }
                          frame True {
                            n524 = case shown="False" w1183 {
                              tunnel: w1187 -> [w1189 w1194]
                              tunnel: [w1189 w1194] -> w1186
                              tunnel: w1185 -> [w1188 w1195]
                              tunnel: [w1193 w1199] -> w1184
                              frame False {
                                n525 = Unbundle By Name(w1188) -> ("V1 time"=w1190:dbl)
                                n526 = Multiply(x=w1190, y=1000.0) -> (x*y=w1191:dbl)
                                n527 = Greater Or Equal?(x=w1189, y=w1191) -> (x >= y?=w1193:bool)
                              }
                              frame True {
                                n528 = Unbundle By Name(w1195) -> ("V off time"=w1196:dbl)
                                n529 = Multiply(x=w1196, y=1000.0) -> (x*y=w1197:dbl)
                                n530 = Greater Or Equal?(x=w1194, y=w1197) -> (x >= y?=w1199:bool)
                              }
                            }
                          }
                        }
                      }
                      frame "Read", Default {
                        n531 = Unbundle By Name(w1201) -> ("Start time"=w1200:i32)
                        n532 = property on="Number of scans in kinetic cycle" class="DigNum (strict)"() -> ("Value"=w1211:i32)  [unwired: 2 in, 2 out]
                        n533 = Tick Count (ms)() -> (millisecond timer value=w1209:u32)
                        n534 = Subtract(x=w1209, y=w1200) -> (x-y=w1202:u32)
                        n535 = call "GetDetector.vi"() -> ("xpixels"=w1210:i32)  [unwired: 4 in, 3 out]
                        n536 = Equal?(x=w1212, y=1.0) -> (x = y?=w1205:bool)
                        n537 = stacked-sequence {
                          seq-local: [_ _ _ _ _ _ _ _ _ _ w1246 _] -> [_ _ _ _ _ _ _ _ _ _ _ w1267]
                          seq-local: [_ _ _ _ _ _ _ _ w1231 _ _ _] -> [_ _ _ _ _ _ _ _ _ _ _ w1265]
                          seq-local: [_ _ _ _ _ _ _ _ _ _ w1245 _] -> [_ _ _ _ _ _ _ _ _ _ _ w1266]
                          tunnel: [_ _ _ _ _ _ _ _ _ _ _ w1260] -> w1204
                          tunnel: [_ _ _ _ _ _ _ _ _ _ _ w1261] -> w1203
                          tunnel: w1211 -> [_ _ _ _ _ w1224 _ _ _ _ w1242 w1259]
                          tunnel: w1202 -> [_ _ _ _ _ _ _ _ _ _ _ w1262]
                          tunnel: w1210 -> [_ w1217 _ _ _ _ _ _ _ _ _ _]
                          tunnel: w1200 -> [_ _ _ _ _ _ _ _ w1230 _ w1244 _]
                          tunnel: w1208 -> [_ _ _ _ _ _ _ _ _ _ _ w1258]
                          tunnel: w1207 -> [_ _ _ _ _ _ _ _ _ _ _ w1257]
                          tunnel: w1206 -> [_ _ _ _ _ _ _ _ _ _ _ w1256]
                          tunnel: w1205 -> [_ _ _ _ _ _ _ _ _ _ _ w1255]
                          frame #0 {
                            w1216 = u16 3  # AcquisitionMode
                            n538 = call "SetAcquisitionMode.vi"("mode"=w1216) -> ()  [unwired: 1 in, 2 out]
                          }
                          frame #1 {
                            w1218 = u16 0  # ReadMode
                            n539 = property on="xpixels" class="DigNum (strict)"("Value"=w1217) -> ()  [unwired: 2 in, 2 out]
                            n540 = call "SetReadMode.vi"("mode"=w1218) -> ()  [unwired: 1 in, 2 out]
                          }
                          frame #2 {
                            n541 = call "SetTriggerMode.vi"("mode"=TriggerMode_mode_typedef."Internal") -> ()  [unwired: 1 in, 2 out]
                          }
                          frame #3 {
                            n542 = property on="Exposure time (s)" class="DigNum (strict)"() -> ("Value"=w1220:dbl)  [unwired: 2 in, 2 out]
                            n543 = call "SetExposureTime.vi"("time"=w1220) -> ()  [unwired: 1 in, 2 out]
                          }
                          frame #4 {
                            n544 = call "GetNumberVSSpeeds.vi"() -> ("number"=w1223:i32)  [unwired: 3 in, 2 out]
                            n545 = Subtract(x=w1223, y=1) -> (x-y=w1221:i32)
                            n546 = call "SetVSSpeed.vi"("index"=w1221) -> ()  [unwired: 1 in, 2 out]
                          }
                          frame #5 {
                            n547 = call "SetNumberKinetics.vi"("number"=w1224) -> ()  [unwired: 1 in, 2 out]
                          }
                          frame #6 {
                            w1227 = 0  # Auto Shutter
                            n548 = call "SetShutter.vi"("type"="Shutter opens on TTL", "mode"=w1227, "closingtime"="Shutter open and close time", "openingtime"="Shutter open and close time") -> ()  [unwired: 10 in, 2 out]
                          }
                          frame #7 {
                            # "Meybe delete the exposure time insupt here"
                            n549 = property on="Exposure time (s)" class="DigNum (strict)"() -> ("Value"=w1228:dbl)  [unwired: 2 in, 2 out]
                            n550 = call "GetAcquisitionTimings.vi"("exposure input"=w1228) -> ("exposure"=w1229:sgl)  [unwired: 10 in, 4 out]
                            n551 = property on="Calculated exposure time" class="DigNum (strict)"("Value"=w1229) -> ()  [unwired: 2 in, 2 out]
                          }
                          frame #8 {
                            n552 = flat-sequence {
                              tunnel: [w1233] -> w1231
                              tunnel: w1230 -> [w1232]
                              frame #0 {
                                n553 = Tick Count (ms)() -> (millisecond timer value=w1234:u32)
                                n554 = Subtract(x=w1234, y=w1232) -> (x-y=w1233:u32)
                                "Time before the start of current aquisition (ms)" <- w1233
                              }
                              frame #1 {
                                n555 = call "StartAcquisition.vi"() -> ("DLL error code"=w1235:u32)  [unwired: 2 in, 1 out]
                                n556 = property on="Start Aquisition return code" class="DigNum (strict)"("Value"=w1235) -> ()  [unwired: 2 in, 2 out]
                              }
                            }
                          }
                          frame #9 {
                            n557 = while {
                              stop <- w1239 continue-if-true
                              w1240 = u16 72  # DRV ACQUIRING
                              n558 = call "GetStatus.vi"() -> ("DLL error code"=w1237:u32, "status"=w1238:T19)  [unwired: 3 in, 1 out]
                              n559 = property on="Get status return code" class="DigNum (strict)"("Value"=w1237) -> ()  [unwired: 2 in, 2 out]
                              n560 = Equal?(x=w1238, y=w1240) -> (x = y?=w1239:bool)
                              "IDus not in read loop? (kinetic)" <- FALSE
                            }
                          }
                          frame #10 {
                            n561 = flat-sequence {
                              tunnel: [w1247] -> w1245
                              tunnel: w1244 -> [w1248]
                              tunnel: [w1254] -> w1246
                              tunnel: w1243 -> [w1250]
                              frame #0 {
                                n562 = Tick Count (ms)() -> (millisecond timer value=w1249:u32)
                                n563 = Subtract(x=w1249, y=w1248) -> (x-y=w1247:u32)
                                "Time  after the aquisition (before fetch data), (ms)" <- w1247
                              }
                              frame #1 {
                                n564 = call "GetAcquiredData.vi"("size"=w1250) -> ("DLL error code"=w1251:u32, "array"=w1254:i32[])  [unwired: 2 in, 1 out]
                                n565 = Equal?(x=20002 ("DRV_SUCCESS"), y=w1251) -> (x = y?=→"Get aqisition ok? (kinetic mode)":bool)
                                n566 = property on="get aquired data return code" class="DigNum (strict)"("Value"=w1251) -> ()  [unwired: 2 in, 2 out]
                              }
                            }
                            n567 = Multiply(x=1024, y=w1242) -> (x*y=w1243:i32)
                          }
                          frame #11 {
                            n568 = Subtract(x=w1266, y=w1265) -> (x-y=w1264:u32)
                            n569 = Divide(x=w1264, y=w1259) -> (x/y=w1263:dbl)
                            n570 = for {
                              N: w1259 -> [_]
                              tunnel: w1267 -> [w1285]
                              tunnel: w1263 -> [w1283]
                              tunnel: w1262 -> [w1280]
                              shift-right: [w1278] -> w1260
                              shift-left: w1256 -> [w1277]
                              shift-right: [w1270] -> w1261
                              shift-left: w1258 -> [w1275]
                              tunnel: w1257 -> [w1273]
                              tunnel: w1255 -> [w1271]
                              i -> [w1269]
                              w1279 = 1024 ("x")
                              n571 = Equal To 0?(x=w1269) -> (x = 0?=w1268:bool)
                              n572 = Multiply(x=w1269, y=w1283) -> (x*y=w1282:dbl)
                              n573 = Multiply(x=w1279, y=w1269) -> (x*y=w1284:i32)
                              n574 = Add(x=w1282, y=w1280) -> (x+y=w1276:dbl)
                              n575 = Array Subset(array=w1285, index=w1284, length=w1279) -> (w1281:i32[])
                              n576 = And(x=w1268, y=w1271) -> (x .and. y?=w1272:bool)
                              n577 = And(x=w1273, y=w1272) -> (x .and. y?=w1274:bool)
                              n578 = case shown="False" w1274 {
                                tunnel: w1281 -> [w1286 w1299]
                                tunnel: [w1291 w1302] -> w1278
                                tunnel: w1277 -> [w1292 _]
                                tunnel: w1276 -> [w1289 w1304]
                                tunnel: [w1288 w1303] -> w1270
                                tunnel: w1275 -> [w1290 _]
                                tunnel: w1268 -> [w1287 _]
                                frame False {
                                n579 = case shown="True" w1287 {
                                tunnel: w1286 -> [_ w1295]
                                frame False {
                                }
                                frame True {
                                n580 = for {
                                N: 1023 -> [_]
                                tunnel: [w1297] -> _ mode=indexing
                                tunnel: [w1297] -> w1294 mode=indexing
                                i -> [w1298]
                                n581 = Increment(x=w1298) -> (x+1=w1297:i32)
                                }
                                n582 = Bundle(w1294, w1295) -> (w1293:cluster{i32[], i32[]})  [unwired: 1 in]
                                n583 = property class="XYGraph (strict)"("Value"=w1293) -> ()  [unwired: 2 in, 2 out]
                                }
                                }
                                n584 = Build Array (concatenate)(w1292, w1286) -> (w1291:dbl[][])
                                n585 = Build Array (concatenate)(w1290, w1289) -> (w1288:dbl[])
                                }
                                frame True {
                                n586 = for {
                                N: 1023 -> [_]
                                tunnel: [w1306] -> w1300 mode=indexing
                                i -> [w1307]
                                n587 = Increment(x=w1307) -> (x+1=w1306:i32)
                                }
                                n588 = Bundle(w1300, w1299) -> (w1301:cluster{i32[], i32[]})  [unwired: 1 in]
                                n589 = Build Array(w1304) -> (w1303:dbl[])
                                n590 = Build Array(w1300, w1299) -> (w1302:i32[][])
                                n591 = property class="XYGraph (strict)"("Value"=w1301) -> ()  [unwired: 2 in, 2 out]
                                }
                              }
                            }
                          }
                        }
                      }
                      frame "Wait" {
                        w1312 = 1000.0 ("y")
                        n592 = Unbundle By Name(w1315) -> ("Sample rate"=w1314:dbl)
                        n593 = property on="Slow sample time (s)" class="DigNum (strict)"() -> ("Value"=w1311:dbl)  [unwired: 2 in, 2 out]
                        n594 = Multiply(x=w1312, y=w1311) -> (x*y=w1310:dbl)
                        n595 = Greater?(x=w1309, y=w1310) -> (0:w1308:bool)
                        n596 = case shown="True" w1308 {
                          tunnel: w1314 -> [_ w1320]
                          tunnel: w1312 -> [_ w1319]
                          frame False {
                          }
                          frame True {
                            n597 = Multiply(x=w1320, y=w1319) -> (x*y=w1321:dbl)
                            n598 = Wait (ms)(milliseconds to wait=w1321) -> ()  [unwired: 1 out]
                          }
                        }
                      }
                    }
                    n599 = case shown="True" w1154 {
                      frame False {
                      }
                      frame True {
                        n600 = property on="IDus not in read loop? (kinetic)" class="Bool (strict)"("Value"=TRUE ("IDus not in read loop? (kinetic)")) -> ()  [unwired: 2 in, 2 out]
                      }
                    }
                  }
                }
              }
              n601 = Bundle By Name(cluster=w960, "Time for spectrum measurment"=w983, "Time elapsed"=w985, "Spectrum"=w984) -> (w980:T11)
              n602 = Bundle By Name(cluster=w980, "Time for I measurment"=w982, "Current array"=w968) -> (w981:T11)
              n603 = local read "V (during measurment)"() -> (w987:dbl)
              n604 = property on="V2 applied?" class="Bool (strict)"() -> ("Value"=w967:bool)  [unwired: 2 in, 2 out]
              n605 = Unbundle By Name(w980) -> ("V 1"=w988:dbl)
              n606 = Equal?(x=w988, y=w987) -> (x = y?=w989:bool)
              n607 = And(x=w967, y="Square wave?") -> (x .and. y?=w966:bool)
              n608 = case shown="True" w989 {
                tunnel: [w1501 w1506] -> w990
                tunnel: w966 -> [_ w1505]
                tunnel: "Square wave?" -> [w1500 w1504]
                frame False {
                  n609 = case shown="True" w1500 {
                    tunnel: [OSSPEC."Read Potential and spectrum" OSSPEC."Apply V1"] -> w1501
                    frame False {
                    }
                    frame True {
                    }
                  }
                }
                frame True {
                  n610 = case shown="False" w1505 {
                    tunnel: [OSSPEC."Apply V2" OSSPEC."End measurment"] -> w1506
                    tunnel: w1504 -> [_ _]
                    frame False {
                    }
                    frame True {
                    }
                  }
                }
              }
            }
            frame "Reinitialise Cell" {
              # "this state is no longer used as it adds a 1-300 ms delay before the spectrum is measured as the mode is shifted"
              n611 = flat-sequence {
                tunnel: w1515 -> [w1519]
                tunnel: [w1518] -> w1510
                tunnel: w1510 -> [w1522]
                tunnel: [w1521] -> w1509
                tunnel: [w1523] -> w1514
                tunnel: w1509 -> [w1523]
                frame #0 {
                  n612 = To Long Integer(number=T17."IStat4EL" ("Configuration")) -> (32bit integer=w1517:i32)
                  n613 = call "IV setconnectionmode.vi"("error in (no error)"=w1519, "value"=w1517) -> ("error out"=w1518:errorcluster)  [unwired: 7 in, 2 out]
                }
                frame #1 {
                  n614 = call "IV setcurrent.vi"("error in (no error)"=w1522, "value"=0.0) -> ("error out"=w1521:errorcluster)  [unwired: 7 in, 2 out]
                }
                frame #2 {
                }
              }
              n615 = Unbundle By Name(w1511) -> ()  [unwired: 3 out]
            }
            frame "Apply V1" {
              n616 = property on="Use autolab?" class="Bool (strict)"() -> ("Value"=w1527:bool)  [unwired: 2 in, 2 out]
              n617 = property on="Potential  During PD" class="WFChart (strict)"("History Data"=dbl[] []) -> ()  [unwired: 2 in, 2 out]
              n618 = property on="Current during PD" class="WFChart (strict)"("History Data"=dbl[] []) -> ()  [unwired: 2 in, 2 out]
              n619 = flat-sequence {
                tunnel: w1535 -> [w1541]
                tunnel: w1534 -> [w1540]
                tunnel: [w1539] -> w1529
                tunnel: [w1538] -> w1528
                tunnel: w1527 -> [w1537]
                tunnel: [w1536] -> w1526
                tunnel: w1535 -> [w1582]
                tunnel: w1529 -> [w1580]
                tunnel: [w1581] -> w1531
                tunnel: [w1576] -> w1530
                tunnel: w1528 -> [w1575]
                tunnel: w1527 -> [w1574]
                tunnel: w1526 -> [w1573]
                frame #0 {
                  n620 = case shown="True" w1537 {
                    tunnel: w1541 -> [w1547 w1564]
                    tunnel: w1540 -> [w1546 _]
                    tunnel: [w1545 w1556] -> w1539
                    tunnel: [w1543 w1563] -> w1538
                    tunnel: [refnum<k24> refnum ("Value") w1560] -> w1536
                    frame False {
                      n621 = Unbundle By Name(w1547) -> ("V 1"=w1545:dbl)
                      n622 = Absolute Value(x=w1545) -> (abs(x)=w1549:dbl)
                      n623 = local write "V (during measurment)"(w1545) -> ()
                      n624 = Greater?(x=w1549, y=3.0) -> (0:w1548:bool)
                      n625 = case shown="False" w1548 {
                        tunnel: [w1550 w1552] -> w1543
                        tunnel: w1546 -> [w1550 w1551]
                        frame False {
                        }
                        frame True {
                          # "abort if E >3 V"
                          n626 = call "IV setcellon.vi"("error in (no error)"=w1551, "cellon"=0) -> ("error out"=w1554:errorcluster)  [unwired: 7 in, 2 out]
                          n627 = call "IV close.vi"("error in (no error)"=w1554) -> ("error out"=w1552:errorcluster)  [unwired: 9 in, 1 out]
                          n628 = call "Display Message to User3"("error in (no error)"=w1552) -> ("OK"=w1555:bool)  [unwired: 9 in, 1 out]
                          n629 = Stop(stop? (T)=w1555) -> ()
                        }
                      }
                    }
                    frame True {
                      w1570 = 1 items=["Off", "On"] ("CellOnOff")
                      n630 = property on="Ei" class="Ref (strict)"() -> ("Value"=w1560:refnum<k24>)  [unwired: 2 in, 2 out]
                      n631 = property on="Sampler 2" class="Ref (strict)"() -> ("Value"=w1566:refnum<k24>)  [unwired: 2 in, 2 out]
                      n632 = property class="EI" props=["EiStatusSupportedFor"](reference=w1560) -> (error out=w1562:errorcluster)  [unwired: 1 in, 2 out]
                      n633 = property class="EI" props=["Bandwidth", "CurrentRange", "Mode", "Potential", "Current"](reference=w1560) -> (error out=w1568:errorcluster, "Potential"=w1572:dbl, "Current"=w1571:dbl)  [unwired: 1 in, 4 out]
                      n634 = invoke class="Sampler" method="Sample"(reference=w1566) -> (error out=w1561:errorcluster)  [unwired: 2 in, 2 out]
                      n635 = Unbundle By Name(w1564) -> ("V 1"=w1556:dbl)
                      n636 = call "Range_selector.vi"("potential"=w1572, "current"=w1571) -> ("range integer"=w1569:i32)  [unwired: 9 in]
                      n637 = property class="EI"(reference=w1560, error in=w1568, "CellOnOff"=w1570, "CurrentRange"=w1569) -> (error out=w1567:errorcluster)  [unwired: 1 out]
                      n638 = call "P_Stat_Status1.vi"("error in (no error)"=w1567, ".NET Refnum in"=w1560) -> ("error out"=w1565:errorcluster, "PotentialOverload"=w1557:bool, "CurrentOverload"=w1559:bool, "Cell"=w1558:bool)  [unwired: 3 in, 3 out]
                      n639 = Merge Errors(w1565, w1562, w1561) -> (w1563:errorcluster)
                      n640 = property on="V (during measurment)" class="DigNum (strict)"("Value"=w1556) -> ()  [unwired: 2 in, 2 out]
                      n641 = property on="Cell on?" class="Bool (strict)"("Value"=w1558) -> ()  [unwired: 2 in, 2 out]
                      n642 = property on="PotentialOverload" class="Bool (strict)"("Value"=w1557) -> ()  [unwired: 2 in, 2 out]
                      n643 = property on="CurrentOverload" class="Bool (strict)"("Value"=w1559) -> ()  [unwired: 2 in, 2 out]
                    }
                  }
                }
                frame #1 {
                  n644 = property on="Square wave?" class="Bool (strict)"() -> ("Value"=w1578:bool)  [unwired: 2 in, 2 out]
                  n645 = property on="V2 applied?" class="Bool (strict)"() -> ("Value"=w1579:bool)  [unwired: 2 in, 2 out]
                  n646 = case shown="True" w1574 {
                    tunnel: w1580 -> [w1585 w1588]
                    tunnel: [w1584 w1587] -> w1576
                    tunnel: w1575 -> [w1583 w1589]
                    tunnel: w1573 -> [_ w1586]
                    frame False {
                      n647 = call "IV setpotential.vi"("error in (no error)"=w1583, "value"=w1585) -> ("error out"=w1584:errorcluster)  [unwired: 7 in, 2 out]
                    }
                    frame True {
                      n648 = property class="EI"(reference=w1586, error in=w1589, "Setpoint"=w1588) -> (error out=w1587:errorcluster)  [unwired: 1 out]
                    }
                  }
                  n649 = And(x=w1578, y=w1579) -> (x .and. y?=w1577:bool)
                  n650 = case shown="False" w1577 {
                    tunnel: w1582 -> [w1593 w1594]
                    tunnel: [w1592 w1594] -> w1581
                    frame False {
                      n651 = Tick Count (ms)() -> (millisecond timer value=w1590:u32)
                      n652 = Bundle By Name(cluster=w1593, "Start time"=w1590, "Time elapsed"=0) -> (w1592:T11)
                    }
                    frame True {
                    }
                  }
                }
              }
            }
            frame "Apply V2" {
              n653 = Tick Count (ms)() -> (millisecond timer value=w1602:u32)
              n654 = flat-sequence {
                tunnel: w1597 -> [w1615]
                tunnel: [w1616] -> w1608
                tunnel: w1607 -> [w1614]
                tunnel: [w1609] -> w1604
                tunnel: [w1613] -> w1603
                tunnel: w1602 -> [w1613]
                tunnel: w1597 -> [w1612]
                tunnel: [w1611] -> w1596
                tunnel: [w1610] -> w1595
                tunnel: w1608 -> [w1652]
                tunnel: w1604 -> [w1651]
                tunnel: w1603 -> [w1650]
                tunnel: [w1650] -> w1600
                tunnel: [w1649] -> w1598
                tunnel: w1596 -> [w1647]
                tunnel: w1595 -> [w1646]
                frame #0 {
                  n655 = property on="Use autolab?" class="Bool (strict)"() -> ("Value"=w1611:bool)  [unwired: 2 in, 2 out]
                  n656 = Unbundle By Name(w1615) -> ("V 2"=w1609:dbl)
                  n657 = Absolute Value(x=w1609) -> (abs(x)=w1619:dbl)
                  n658 = Greater?(x=w1619, y=3.0) -> (0:w1617:bool)
                  n659 = local write "V (during measurment)"(w1609) -> ()
                  n660 = case shown="True" w1611 {
                    tunnel: w1617 -> [w1623 _]
                    tunnel: [w1622 w1637] -> w1616
                    tunnel: w1614 -> [w1621 _]
                    tunnel: w1612 -> [_ _]
                    tunnel: [refnum<k24> refnum ("Value") w1636] -> w1610
                    tunnel: w1609 -> [_ w1634]
                    frame False {
                      n661 = case shown="True" w1623 {
                        tunnel: [w1624 w1626] -> w1622
                        tunnel: w1621 -> [w1624 w1625]
                        frame False {
                        }
                        frame True {
                          # "abort if E >3 V"
                          n662 = call "IV setcellon.vi"("error in (no error)"=w1625, "cellon"=0) -> ("error out"=w1628:errorcluster)  [unwired: 7 in, 2 out]
                          n663 = call "IV close.vi"("error in (no error)"=w1628) -> ("error out"=w1626:errorcluster)  [unwired: 9 in, 1 out]
                          n664 = call "Display Message to User4"("error in (no error)"=w1626) -> ("OK"=w1629:bool)  [unwired: 9 in, 1 out]
                          n665 = Stop(stop? (T)=w1629) -> ()
                        }
                      }
                    }
                    frame True {
                      w1630 = -2 items=["CR07_1A"=0, "CR06_10A"=1, "CR01_100A"=2, "CR00_1000A"=3, "CR05_20A"=20, "CR04_40A"=40, "CR03_50A"=60, "CR02_80A"=80, "CR19_1pA"=-12, "CR18_10pA"=-11, "CR17_100pA"=-10, "CR16_1nA"=-9, "CR15_10nA"=-8, "CR14_100nA"=-7, "CR13_1uA"=-6, "CR12_10uA"=-5, "CR11_100uA"=-4, "CR10_1mA"=-3, "CR09_10mA"=-2, "CR08_100mA"=-1] ("CurrentRange")
                      w1643 = 1 items=["Off", "On"] ("CellOnOff")
                      n666 = property on="Ei" class="Ref (strict)"() -> ("Value"=w1636:refnum<k24>)  [unwired: 2 in, 2 out]
                      n667 = property on="Sampler 2" class="Ref (strict)"() -> ("Value"=w1638:refnum<k24>)  [unwired: 2 in, 2 out]
                      n668 = property class="EI"(reference=w1636) -> (error out=w1635:errorcluster, "EiStatusSupportedFor"=w1633:string[])  [unwired: 1 in, 1 out]
                      n669 = property class="EI" props=["Bandwidth", "CurrentRange", "Mode", "Potential", "Current"](reference=w1636) -> (error out=w1642:errorcluster, "Potential"=w1645:dbl, "Current"=w1644:dbl)  [unwired: 1 in, 4 out]
                      n670 = invoke class="Sampler" method="Sample"(reference=w1638) -> (error out=w1639:errorcluster)  [unwired: 2 in, 2 out]
                      n671 = call "Range_selector.vi"("potential"=w1645, "current"=w1644) -> ()  [unwired: 9 in, 1 out]
                      n672 = property on="EI status supported for" class="Arr (strict)"("Value"=w1633) -> ()  [unwired: 2 in, 2 out]
                      n673 = property class="EI"(reference=w1636, error in=w1642, "CellOnOff"=w1643, "CurrentRange"=w1630, "Setpoint"=w1634) -> (error out=w1641:errorcluster)  [unwired: 1 out]
                      n674 = property on="CurrentRange" class="DigNum (strict)"("Value"=w1630) -> ()  [unwired: 2 in, 2 out]
                      n675 = call "P_Stat_Status1.vi"("error in (no error)"=w1641, ".NET Refnum in"=w1636) -> ("error out"=w1640:errorcluster, "PotentialOverload"=w1631:bool, "CurrentOverload"=w1632:bool)  [unwired: 3 in, 4 out]
                      n676 = property on="CurrentOverload" class="Bool (strict)"("Value"=w1632) -> ()  [unwired: 2 in, 2 out]
                      n677 = Merge Errors(w1640, w1635, w1639) -> (w1637:errorcluster)
                      n678 = property on="PotentialOverload" class="Bool (strict)"("Value"=w1631) -> ()  [unwired: 2 in, 2 out]
                    }
                  }
                }
                frame #1 {
                  n679 = case shown="False" w1647 {
                    tunnel: w1652 -> [w1655 w1658]
                    tunnel: w1651 -> [w1654 w1656]
                    tunnel: [w1653 w1657] -> w1649
                    tunnel: w1646 -> [_ w1659]
                    frame False {
                      n680 = call "IV setpotential.vi"("error in (no error)"=w1655, "value"=w1654) -> ("error out"=w1653:errorcluster)  [unwired: 7 in, 2 out]
                    }
                    frame True {
                      n681 = property class="EI"(reference=w1659, error in=w1658, "Setpoint"=w1656) -> (error out=w1657:errorcluster)  [unwired: 1 out]
                    }
                  }
                  "V2 applied?" <- TRUE ("V2 applied")
                }
              }
              n682 = Tick Count (ms)() -> (millisecond timer value=w1599:u32)
              n683 = Subtract(x=w1599, y=w1600) -> (x-y=→"Time taken to apply V2":u32)
              n684 = Unbundle By Name(w1597) -> ()  [unwired: 3 out]
            }
            frame "End measurment" {
              w1671 = ext 0.00099999999999999999996
              w1688 = TRUE
              n685 = Unbundle By Name(w1661) -> ("Time for spectrum measurment"=w1667:i32[], "Spectrum"=w1684:dbl[][])
              n686 = Unbundle By Name(w1661) -> ("Current array"=w1678:dbl[], "Time for I measurment"=w1673:i32[])
              n687 = Unbundle By Name(w1661) -> ("Time for E measurment"=w1670:i32[], "Potential array"=w1679:dbl[])
              n688 = Multiply(x=w1667, y=ext 0.00099999999999999999996) -> (x*y=w1666:ext[])
              n689 = Multiply(x=w1673, y=w1671) -> (x*y=w1672:ext[])
              n690 = Multiply(x=w1671, y=w1670) -> (x*y=w1669:ext[])
              n691 = Build Array(w1672, w1678) -> (w1677:ext[][])
              n692 = Build Array(w1669, w1679) -> (w1675:ext[][])
              n693 = Insert Into Array(array=w1666, index=0, new element=0 ("new element/subarray")) -> (w1682:ext[])
              n694 = Transpose 2D Array(2D array=w1677) -> (transposed array=w1676:ext[][])
              n695 = Transpose 2D Array(2D array=w1675) -> (transposed array=w1674:ext[][])
              n696 = Insert Into Array(array=w1684, index (col)=0 ("disabled index (col)"), new element=w1682) -> (w1681:dbl[][])  [unwired: 1 in]
              n697 = call "Write-OSP-J-t.vi"("Init cluster"=w1661, "Array"=w1676) -> ()  [unwired: 10 in]
              n698 = call "Write-OSP-E-t.vi"("Init cluster"=w1661, "Array"=w1674) -> ()  [unwired: 10 in]
              n699 = Transpose 2D Array(2D array=w1681) -> (transposed array=w1680:dbl[][])
              n700 = call "Write-OSP-SP.vi"("Init cluster"=w1661, "Array"=w1680) -> ()  [unwired: 10 in]
              n701 = property on="T reached?" class="Bool (strict)"("Value"=FALSE ("T reached?")) -> ()  [unwired: 2 in, 2 out]
              n702 = Unbundle By Name(w1661) -> ("Default\n potential"=w1663:dbl)
              n703 = property on="Use autolab?" class="Bool (strict)"() -> ("Value"=w1664:bool)  [unwired: 2 in, 2 out]
              n704 = case shown="True" w1664 {
                tunnel: w1663 -> [w1692 w1708]
                tunnel: w1689 -> [w1691 w1707]
                tunnel: [w1690 w1706] -> w1687
                frame False {
                  n705 = flat-sequence {
                    tunnel: w1691 -> [w1696]
                    tunnel: [w1695] -> w1694
                    tunnel: w1692 -> [w1701]
                    tunnel: w1694 -> [w1700]
                    tunnel: [w1699] -> w1693
                    tunnel: w1693 -> [w1703]
                    tunnel: [w1702] -> w1690
                    frame #0 {
                      n706 = To Long Integer(number=T17."EStat4EL" ("Configuration")) -> (32bit integer=w1698:i32)
                      n707 = call "IV setconnectionmode.vi"("error in (no error)"=w1696, "value"=w1698) -> ("error out"=w1695:errorcluster)  [unwired: 7 in, 2 out]
                    }
                    frame #1 {
                      n708 = call "IV setpotential.vi"("error in (no error)"=w1700, "value"=w1701) -> ("error out"=w1699:errorcluster)  [unwired: 7 in, 2 out]
                    }
                    frame #2 {
                      n709 = call "IV getcurrent.vi"("error in (no error)"=w1703) -> ("error out"=w1702:errorcluster, "value out"=w1704:dbl)  [unwired: 8 in, 1 out]
                      n710 = call "Current ranging routine (SubVI).vi"("Current"=w1704) -> ()  [unwired: 11 in]
                    }
                  }
                }
                frame True {
                  w1713 = 0 items=["Off", "On"] ("CellOnOff")
                  n711 = property on="Ei" class="Ref (strict)"() -> ("Value"=w1705:refnum<k24>)  [unwired: 2 in, 2 out]
                  n712 = disable-structure shown="Enabled" {
                    disable-tunnel: [w1733 _] -> w1711
                    disable-tunnel: [w1732 _] -> w1710
                    disable-tunnel: [w1731 -3 ("range integer")] -> w1709
                    disable-tunnel: w1708 -> [w1729 _]
                    disable-tunnel: w1707 -> [w1727 _]
                    disable-tunnel: w1705 -> [w1722 _]
                    frame Disabled {
                      w1728 = -2 items=["CR07_1A"=0, "CR06_10A"=1, "CR01_100A"=2, "CR00_1000A"=3, "CR05_20A"=20, "CR04_40A"=40, "CR03_50A"=60, "CR02_80A"=80, "CR19_1pA"=-12, "CR18_10pA"=-11, "CR17_100pA"=-10, "CR16_1nA"=-9, "CR15_10nA"=-8, "CR14_100nA"=-7, "CR13_1uA"=-6, "CR12_10uA"=-5, "CR11_100uA"=-4, "CR10_1mA"=-3, "CR09_10mA"=-2, "CR08_100mA"=-1] ("CurrentRange")
                      w1730 = 0 items=["Potentiostatic", "Galvanostatic"] ("Mode")
                      n713 = property class="EI"(reference=w1722, error in=w1727, "Setpoint"=w1729, "Mode"=w1730, "CurrentRange"=w1728) -> (error out=w1724:errorcluster)  [unwired: 1 out]
                      n714 = property on="Sampler 2" class="Ref (strict)"() -> ("Value"=w1723:refnum<k24>)  [unwired: 2 in, 2 out]
                      n715 = property class="EI"(reference=w1722, error in=w1724) -> ("Current"=w1725:dbl, "Potential"=w1726:dbl)  [unwired: 2 out]
                      n716 = property class="EI" props=["EiStatusSupportedFor"](reference=w1722) -> (error out=w1733:errorcluster)  [unwired: 1 in, 2 out]
                      n717 = invoke class="Sampler" method="Sample"(reference=w1723) -> (error out=w1732:errorcluster)  [unwired: 2 in, 2 out]
                      n718 = flat-sequence {
                        tunnel: [w1737] -> w1731
                        tunnel: w1726 -> [w1736]
                        tunnel: w1725 -> [w1735]
                        frame #0 {
                          n719 = Wait (ms)(milliseconds to wait=u32 50) -> ()  [unwired: 1 out]
                        }
                        frame #1 {
                          n720 = call "Range_selector.vi"("potential"=w1736, "current"=w1735) -> ("range integer"=w1737:i32)  [unwired: 9 in]
                        }
                      }
                    }
                    frame Enabled {
                    }
                  }
                  n721 = property class="EI"(reference=w1705, "CellOnOff"=w1713, "CurrentRange"=w1709) -> (error out=w1712:errorcluster)  [unwired: 1 in, 1 out]
                  n722 = disable-structure shown="Enabled" {
                    disable-tunnel: w1712 -> [w1721 _]
                    disable-tunnel: w1711 -> [w1719 _]
                    disable-tunnel: w1710 -> [w1718 _]
                    disable-tunnel: [w1717 _] -> w1706
                    disable-tunnel: w1705 -> [w1716 _]
                    frame Disabled {
                      n723 = call "P_Stat_Status1.vi"("error in (no error)"=w1721, ".NET Refnum in"=w1716) -> ("error out"=w1720:errorcluster, "PotentialOverload"=w1715:bool, "CurrentOverload"=w1714:bool)  [unwired: 3 in, 4 out]
                      n724 = property on="CurrentOverload" class="Bool (strict)"("Value"=w1714) -> ()  [unwired: 2 in, 2 out]
                      n725 = Merge Errors(w1720, w1719, w1718) -> (w1717:errorcluster)
                      n726 = property on="PotentialOverload" class="Bool (strict)"("Value"=w1715) -> ()  [unwired: 2 in, 2 out]
                    }
                    frame Enabled {
                    }
                  }
                }
              }
              n727 = property on="V2 applied?" class="Bool (strict)"("Value"=FALSE ("V2 applied?")) -> ()  [unwired: 2 in, 2 out]
              "PD ENDED\nEXIT MEASURMENT" <- w1688
            }
          }
        }
        n728 = property on="PD ENDED\nEXIT MEASURMENT" class="Bool (strict)"() -> ("Value"=w537:bool)  [unwired: 2 in, 2 out]
        n729 = case shown="True" w537 {
          tunnel: [State."Wait for Event" ("f") State."Exit" ("f")] -> w546
          frame False {
          }
          frame True {
          }
        }
      }
      frame "Initialse and cool iDus" {
        # "Also re-intialise constants"
        n730 = Unbundle By Name(w1740) -> ("Return detector to \nroom T"=w1743:bool)
        n731 = case shown="False" w1743 {
          tunnel: [State."Wait for Event" ("f") State."Wait for Event" ("f")] -> w1742
          frame False {
            w1752 = 20002  # DRV_SUCCESS
            n732 = stacked-sequence {
              seq-local: [_ _ _ _ _ _ w1818] -> [_ _ _ _ _ _ _]
              seq-local: [_ _ _ _ _ _ w1819] -> [_ _ _ _ _ _ _]
              tunnel: w1752 -> [w1808 _ _ _ _ _ _]
              tunnel: [w1807 _ _ _ _ _ _] -> w1751
              tunnel: [_ _ _ _ _ _ w1818] -> _
              tunnel: [_ _ _ _ _ _ w1819] -> w1746
              frame #0 {
                n733 = call "Initialize.vi"("directory (\"\")"="" ("directory (\"\")")) -> ("DLL error code"=w1810:u32)  [unwired: 1 in, 1 out]
                "Init. return code" <- w1810
                n734 = Equal?(x=w1808, y=w1810) -> (x = y?=w1807:bool)
              }
              frame #1 {
                n735 = Wait (ms)(milliseconds to wait=u32 2000) -> ()  [unwired: 1 out]
              }
              frame #2 {
                w1812 = u16 0  # ReadMode
                n736 = call "SetReadMode.vi"("mode"=w1812) -> ()  [unwired: 1 in, 2 out]
              }
              frame #3 {
                w1813 = u16 1  # AcquisitionMode
                n737 = call "SetAcquisitionMode.vi"("mode"=w1813) -> ()  [unwired: 1 in, 2 out]
              }
              frame #4 {
                w1814 = 0
                n738 = call "SetHSSpeed.vi"("index"=w1814, "type"=w1814) -> ()  [unwired: 2 in, 2 out]
              }
              frame #5 {
                n739 = call "GetNumberVSSpeeds.vi"() -> ("number"=w1817:i32)  [unwired: 3 in, 2 out]
                n740 = Subtract(x=w1817, y=1) -> (x-y=w1815:i32)
                n741 = call "SetVSSpeed.vi"("index"=w1815) -> ()  [unwired: 1 in, 2 out]
              }
              frame #6 {
                n742 = call "GetDetector.vi"() -> ("ypixels"=w1818:i32, "xpixels"=w1819:i32)  [unwired: 4 in, 2 out]
                "xpixels" <- w1819
                "ypixels" <- w1818
              }
            }
            n743 = flat-sequence {
              tunnel: w1751 -> [w1803]
              tunnel: [w1802] -> w1750
              frame #0 {
                n744 = case shown="False" w1803 {
                  selector: w1803 -> [w1805 w1806]
                  tunnel: [w1804 w1806] -> w1802
                  frame False {
                    n745 = Not(x=w1805) -> (.not. x?=w1804:bool)
                    n746 = call "Display Message to User5"() -> ()  [unwired: 10 in, 2 out]
                    n747 = Stop(stop? (T)=w1804) -> ()
                  }
                  frame True {
                  }
                }
              }
            }
            n748 = flat-sequence {
              tunnel: w1750 -> [w1759]
              tunnel: [w1757] -> w1747
              tunnel: w1746 -> [w1757]
              tunnel: [w1756] -> _
              frame #0 {
                w1760 = 36  # DRV_TEMP_STABILIZED
                w1761 = 20002  # DRV_SUCCESS
                # "set T ok?"
                # "timings ok?"
                n749 = stacked-sequence {
                  seq-local: [_ _ w1764 _ _ _] -> [_ _ _ _ _ _]
                  seq-local: [_ _ _ w1772 _ _] -> [_ _ _ _ w1776 w1777]
                  tunnel: w1761 -> [_ _ w1766 w1775 _ _]
                  tunnel: "Temperature\n(degrees C)" -> [_ _ _ w1773 _ _]
                  tunnel: w1760 -> [_ _ _ _ _ w1778]
                  tunnel: w1759 -> [_ _ w1765 _ _ _]
                  tunnel: [_ _ _ _ _ w1777] -> w1756
                  frame #0 {
                    n750 = call "SetTriggerMode.vi"("mode"=TriggerMode_mode_typedef."Internal") -> ()  [unwired: 1 in, 2 out]
                  }
                  frame #1 {
                    n751 = property on="Exposure time (s)" class="DigNum (strict)"() -> ("Value"=w1763:dbl)  [unwired: 2 in, 2 out]
                    n752 = call "SetExposureTime.vi"("time"=w1763) -> ()  [unwired: 1 in, 2 out]
                  }
                  frame #2 {
                    n753 = case shown="True" w1765 {
                      tunnel: w1766 -> [_ w1770]
                      tunnel: [FALSE w1771] -> w1764
                      frame False {
                      }
                      frame True {
                        n754 = call "GetAcquisitionTimings.vi"() -> ("exposure"=→"Calculated exposure time":sgl, "DLL error code"=w1769:u32)  [unwired: 11 in, 3 out]
                        "Check timings return code" <- w1769
                        n755 = Equal?(x=w1770, y=w1769) -> (x = y?=w1771:bool)
                      }
                    }
                  }
                  frame #3 {
                    n756 = call "SetTemperature.vi"("temperature"=w1773) -> ("DLL error code"=w1774:u32)  [unwired: 1 in, 1 out]
                    "Set temprature\nreturn code" <- w1774
                    n757 = Equal?(x=w1775, y=w1774) -> (x = y?=w1772:bool)
                  }
                  frame #4 {
                    n758 = case shown="True" w1776 {
                      frame False {
                      }
                      frame True {
                        n759 = call "CoolerON.vi"() -> ()  [unwired: 2 in, 2 out]
                      }
                    }
                  }
                  frame #5 {
                    n760 = case shown="True" w1777 {
                      tunnel: w1778 -> [_ w1779]
                      frame False {
                      }
                      frame True {
                        n761 = while {
                          tunnel: w1779 -> [w1783]
                          stop <- w1780 continue-if-true
                          n762 = Wait Until Next ms Multiple(millisecond multiple=u32 500) -> ()  [unwired: 1 out]
                          n763 = call "GetTemperature.vi"() -> ("status"=w1781:T19, "temperature"=→"Curent Temp":i32)  [unwired: 4 in, 2 out]
                          n764 = Not Equal?(x=w1783, y=w1781) -> (x != y?=w1780:bool)
                        }
                      }
                    }
                  }
                }
              }
            }
            n765 = for {
              N: 1023 -> [_]
              tunnel: [w1753] -> w1744 mode=indexing
              i -> [w1755]
              n766 = Add(x=1, y=w1755) -> (x+y=w1753:i32)
            }
            n767 = stacked-sequence {
              seq-local: [w1786 _ _] -> [_ w1791 _]
              tunnel: TRUE -> [w1785 _ _]
              tunnel: w1747 -> [_ _ w1800]
              tunnel: w1744 -> [_ _ w1798]
              frame #0 {
                n768 = case shown="True" w1785 {
                  tunnel: [FALSE w1790] -> w1786
                  frame False {
                  }
                  frame True {
                    w1788 = 20002  # DRV_SUCCESS
                    n769 = call "StartAcquisition.vi"() -> ("DLL error code"=w1789:u32)  [unwired: 2 in, 1 out]
                    "Start Aquisition return code" <- w1789
                    n770 = Equal?(x=w1788, y=w1789) -> (x = y?=w1790:bool)
                  }
                }
              }
              frame #1 {
                n771 = case shown="True" w1791 {
                  frame False {
                  }
                  frame True {
                    n772 = while {
                      stop <- w1794 continue-if-true
                      w1793 = u16 72  # DRV ACQUIRING
                      n773 = call "GetStatus.vi"() -> ("status"=w1792:T19)  [unwired: 3 in, 2 out]
                      n774 = Wait Until Next ms Multiple(millisecond multiple=u32 50) -> ()  [unwired: 1 out]
                      n775 = property on="Get status return code" class="DigNum (strict)"("Value"=w1792) -> ()  [unwired: 2 in, 2 out]
                      n776 = Equal?(x=w1792, y=w1793) -> (x = y?=w1794:bool)
                    }
                  }
                }
              }
              frame #2 {
                n777 = call "GetAcquiredData.vi"("size"=w1800) -> ("DLL error code"=→"get aquired data return code":u32, "array"=w1797:i32[])  [unwired: 2 in, 1 out]
                n778 = Bundle(w1798, "array"=w1797) -> (→"?":cluster{i32[], "array":i32[]})  [unwired: 1 in]
                "T reached?" <- TRUE ("T reached?")
              }
            }
          }
          frame True {
            n779 = property on="T reached?" class="Bool (strict)"("Value"=FALSE ("T reached?")) -> ()  [unwired: 2 in, 2 out]
            n780 = stacked-sequence {
              frame #0 {
                n781 = call "CoolerOFF.vi"() -> ("DLL error code"=→"Cooler Off return code":u32)  [unwired: 2 in, 1 out]
              }
              frame #1 {
                n782 = while {
                  stop <- w1825 continue-if-true
                  n783 = call "GetTemperature.vi"() -> ("temperature"=w1823:i32)  [unwired: 4 in, 3 out]
                  n784 = property on="Curent Temp" class="DigNum (strict)"("Value"=w1823) -> ()  [unwired: 2 in, 2 out]
                  n785 = Less?(x=w1823, y=i16 0) -> (x < y?=w1825:bool)
                  n786 = Wait Until Next ms Multiple(millisecond multiple=u32 500) -> ()  [unwired: 1 out]
                }
              }
              frame #2 {
                n787 = call "ShutDown.vi"() -> ()  [unwired: 2 in, 2 out]
                "Shut down sequence run?" <- TRUE ("Shut down complete?")
              }
            }
          }
        }
      }
    }
    n788 = property on="Use autolab?" class="Bool (strict)"() -> ("Value"=w4:bool)  [unwired: 2 in, 2 out]
    n789 = Equal To 0?(x=w22) -> (x = 0?=w30:bool)
    n790 = case shown="True" w4 {
      tunnel: w31 -> [w47 w83]
      tunnel: w30 -> [w46 _]
      tunnel: [w45 w83] -> w24
      tunnel: [w42 FALSE] -> w20
      frame False {
        n791 = case shown="False" w46 {
          tunnel: w47 -> [w56 w82]
          tunnel: [w55 w80] -> w45
          tunnel: [w50 w74] -> w39
          tunnel: [w51 w75] -> w43
          tunnel: [w53 w81] -> w41
          tunnel: [w49 w73] -> w40
          tunnel: [w52 w76] -> w44
          frame False {
            n792 = call "IV getcellstatus.vi"() -> ("devcellstatus out"=w66:i32)  [unwired: 9 in, 2 out]
            n793 = call "Bitget 8-bits test.vi"("x"=w66) -> ("c"=w62:dbl, "e"=w64:dbl, "f"=w63:dbl, "h"=w65:dbl)  [unwired: 19 in, 4 out]
            n794 = Greater?(x=w62, y=0.0) -> (0:w68:bool)
            n795 = Greater?(x=w64, y=0.0) -> (0:w69:bool)
            n796 = Greater?(x=w63, y=0.0) -> (0:w70:bool)
            n797 = Greater?(x=w65, y=0.0) -> (0:w48:bool)
            n798 = And(x=w66, y=256) -> (x .and. y?=w67:i32)
            n799 = Equal?(x=w67, y=256) -> (x = y?=w71:bool)
            n800 = Bundle By Name(cluster=w56, "I overload"=w68, "Aninput1 overload"=w69, "E overload"=w70, "Cell of button pressed"=w48, "Cell on"=w71) -> (w55:T11)
            n801 = Unbundle By Name(w55) -> ("I overload"=w53:bool, "Aninput1 overload"=w52:bool, "E overload"=w51:bool, "Cell of button pressed"=w50:bool, "Cell on"=w49:bool)
          }
          frame True {
            w72 = FALSE
            # "After closing the driver reset the indicators"
            n802 = property class="XYGraph (strict)"("Value"=cluster{dbl[], dbl[]} {[], []} ("XY Graph")) -> ()  [unwired: 2 in, 2 out]
            n803 = property on="Potentiostat Status" class="Str"("Value"="" ("Device Status indicator")) -> ()  [unwired: 2 in, 2 out]
            n804 = property on="Device serial number" class="Str"("Value"="" ("Device serial number")) -> ()  [unwired: 2 in, 2 out]
            n805 = Bundle By Name(cluster=w82, "I overload"=w72, "Aninput1 overload"=w72, "E overload"=w72, "Cell of button pressed"=w72, "Cell on"=w72) -> (w80:T11)
            n806 = Unbundle By Name(w80) -> ("I overload"=w81:bool, "Aninput1 overload"=w76:bool, "E overload"=w75:bool, "Cell of button pressed"=w74:bool, "Cell on"=w73:bool)
          }
        }
        "I_overload" <- w41
        "Aninput1_overload" <- w44
        "E_overload" <- w43
        "cell-off button pressed" <- w39
        "cell on" <- w40
        n807 = Or(x=w41, y=w43) -> (x .or. y?=w42:bool)
      }
      frame True {
      }
    }
    n808 = Unbundle By Name(w31) -> ("Current"=→"current":dbl, "Serial No"=→"Device serial number":string, "Status"=→"Potentiostat Status":string)
    n809 = Or(x=w25, y=w36) -> (x .or. y?=w35:bool)
    n810 = case shown="False" w20 {
      tunnel: w7 -> [w85 w86]
      tunnel: [w85 w86] -> w21
      frame False {
      }
      frame True {
        n811 = disable-structure shown="Disabled" {
          disable-tunnel: [State."Exit" ("f") _] -> _
          frame Disabled {
            n812 = call "Display Message to User"() -> ()  [unwired: 10 in, 2 out]
          }
          frame Enabled {
          }
        }
      }
    }
  }
